vi "MegaAwesome_12_07_12a_JW.vi"() -> ()   [LabVIEW 2012]
uses:
  data/MegaAwesome_States.ctl
  <vilib>/Utility/inputDevices.llb/keyboardAcquire.vi
  <vilib>/Utility/file.llb/Read From Spreadsheet File (string).vi
  <vilib>/Utility/file.llb/Write To Spreadsheet File (string).vi
panel:
  out "Save Next?":bool
  out "Image Center X":i32
  in  "Disable Flag":bool
  out "Index":string
  in  "Slider Min":dbl=5.0
  in  "Slider Max":dbl=5.0
  out "Opj X Axis":string
  out "X Axis Display Type":string
  in  "Index-Sat":dbl=5.0
  in  "Index-Lin":dbl=5.0
  in  "IndexLog-Lin":dbl=5.0
  in  "IndexLog-Sat":dbl=5.0 caption="Num Pts"
  out "Lin Id-Log Used":dbl[](array[numeric])
  out "Lin-Vg Array-Log Used":dbl[](array[numeric])
  out "Save Array":string[][](array[string])
  out "Folder Index":i32 caption="Length"
  out "Sat Id-Used":dbl[](array[numeric])
  out "Sat Vg Array-Used":dbl[](array[numeric])
  out "Vg Array-Log-Used":dbl[](array[numeric])
  out "Sat Id-Log-Used":dbl[](array[numeric])
  out "Lin Id-Used":dbl[](array[numeric])
  out "Lin-Vg Array-Used":dbl[](array[numeric])
  out "Lin Vd":dbl
  out "Recorded Prop":T1
  out "Current State":T2
  in  "Main Tab Control":T3(tab)
  in  "Transfer File":path
  out "Transfer Folder":path
  in  "Transport\nFolder":path caption="Transport Folder"
  out "Transport\nFile":path caption="Transport File"
  in  "Image Folder":path
  out "Image File":path
  out "Fabrication Prop":T4
  out "Distances":i32[](array[numeric])
  in  "Zoom":i32(slide)=-3 scale=-5.0..5.0
  in  "Magnification":i32(ring) items=["5x", "10x", "20x", "50x", "80x"]
  in  "Undo Button":bool
  in  "Remove Button":bool
  in  "Transfer Plots":T5(tab)=enum."Saturation"
  in  "Lin-Trans Slider":dbl(slide) step=1.0 scale=-40.0..40.0 scale format="%#_1p"
  out "Sqrt-Lin":cluster{dbl[], dbl[]}[](graph)
  in  "Sat-Trans Slider":dbl(slide) step=1.0 scale=-40.0..40.0 scale format="%#_1p"
  out "Sqrt-Sat":cluster{dbl[], dbl[]}[](graph)
  out "Raw- Lin":cluster{dbl[], dbl[]}[](graph)
  out "Raw- Sat":cluster{dbl[], dbl[]}[](graph)
  in  "Log Plots":enum32{"Linear", "Saturation", "Transport"}(tab)=enum."Saturation"
  in  "Lin-Log Slider":dbl(slide) step=1.0 scale=-40.0..40.0 scale format="%#_1p"
  out "Lin-Log":cluster{dbl[], dbl[]}[](graph)
  in  "Sat-Log Slider":dbl(slide) step=1.0 scale=-40.0..40.0 scale format="%#_1p"
  out "Sat-Log":cluster{dbl[], dbl[]}[](graph)
  out "Transport":cluster{ext[], ext[]}[](graph)
  out "Transport Name:":string
  in  "Manual Controls":T6
  in  "File Controls":T7
  out "Date Recorded":string="Date Recorded" caption="Measured"
  out "Data Name:":string
  out "Image Name":string
  out "Date Created":string caption="Fabricated"
  in  "Comments:":string
  out "Rec: Length":dbl caption="Length"
  out "Rec: Width":dbl caption="Width"
  out "Rec: Dielectric (d)":dbl caption="Dielectric (d)" format="%#_3g"
  in  "New: Dielectric":dbl
  in  "New: Length":dbl
  in  "New: Width":dbl
  out "Rec: Temp":dbl caption="Sample Temp" format="%.1f"
  in  "New: Temp":dbl format="%.1f"
  out "Image Out":T8(plugin-control)
  in  "Num Pts":i32=5
  in  "Num Pts Log":i32=5 caption="Num Pts"
  out "Recorded Values Cluster":T9
  out "Calculated Values Cluster":T9 caption="Recorded Values Cluster"
  out "Re-Calculated Values Cluster":T9 caption="Recorded Values Cluster"
  in  "Independant Variable:":string(combo)="Length (um):"
  out "Image Preview":T8(plugin-control)
  out "Total Width":i32
  in  "Index Array":i32(ring) caption="Index" items=["1E", "2E", "2F", "2G", "2H", "3A", "3B", "3C", "3D", "3E", "3F", "3G", "3H", "3J", "4D", "4E", "4F", "4G", "4H", "4J", "5F", "5G", "5H", "6A", "6B", "6F", "6G", "7C", "7D", "7E", "7F", "7G", "8E", "8G", "8H", "9F", "9G", "X 1A", "X 1B", "X 1C", "X 1D", "X 1F", "X 1G", "X 2B", "X 2C", "X 2D"]
  in  "Room Temp":dbl=294.0 caption="Room Temp (K)"
  out "No Image\n File":path=path "\\\\acad1\\physics/Jurchescu-group/JW-PD/Mega Awesome/Image Not Found.png" caption="No Image File"
  out "Origin Project File":path=path "\\\\acad1\\physics/Jurchescu-group/JW-PD/Group Library/Origin Project Files/DeviceData_8_10_12a_JW.opj"
  out "No Transport\n File":path=path "\\\\acad1\\physics/Jurchescu-group/JW-PD/Mega Awesome/No Transport File.txt" caption="No Transport File"
  in  "Transport Style Controls":T10={"Transport Line Size"=1, "Transport Line Color"=16772608} {"Transport Line Size" items=["Extra Small", "Small", "Medium", "Large", "Extra Large"]}
  out "Application Directory":path
  out "Progress":i32(slide) max=46 step=1 scale=0.0..100.0
  # "1)  Select the Transfer File that you would like to analyze:"
  # "Transfer Location"
  # "2) What else would you like to view during your analysis?"
  # "Transport Location"
  # "Image Location"
  # "Recorded"
  # "Calculated"
  # "Re-Calculated"
  # "Manual"
  # "um"
  # "V"
  # "V"
  # "V"
  # "Default File Choices"
  # "Default Analysis Values"
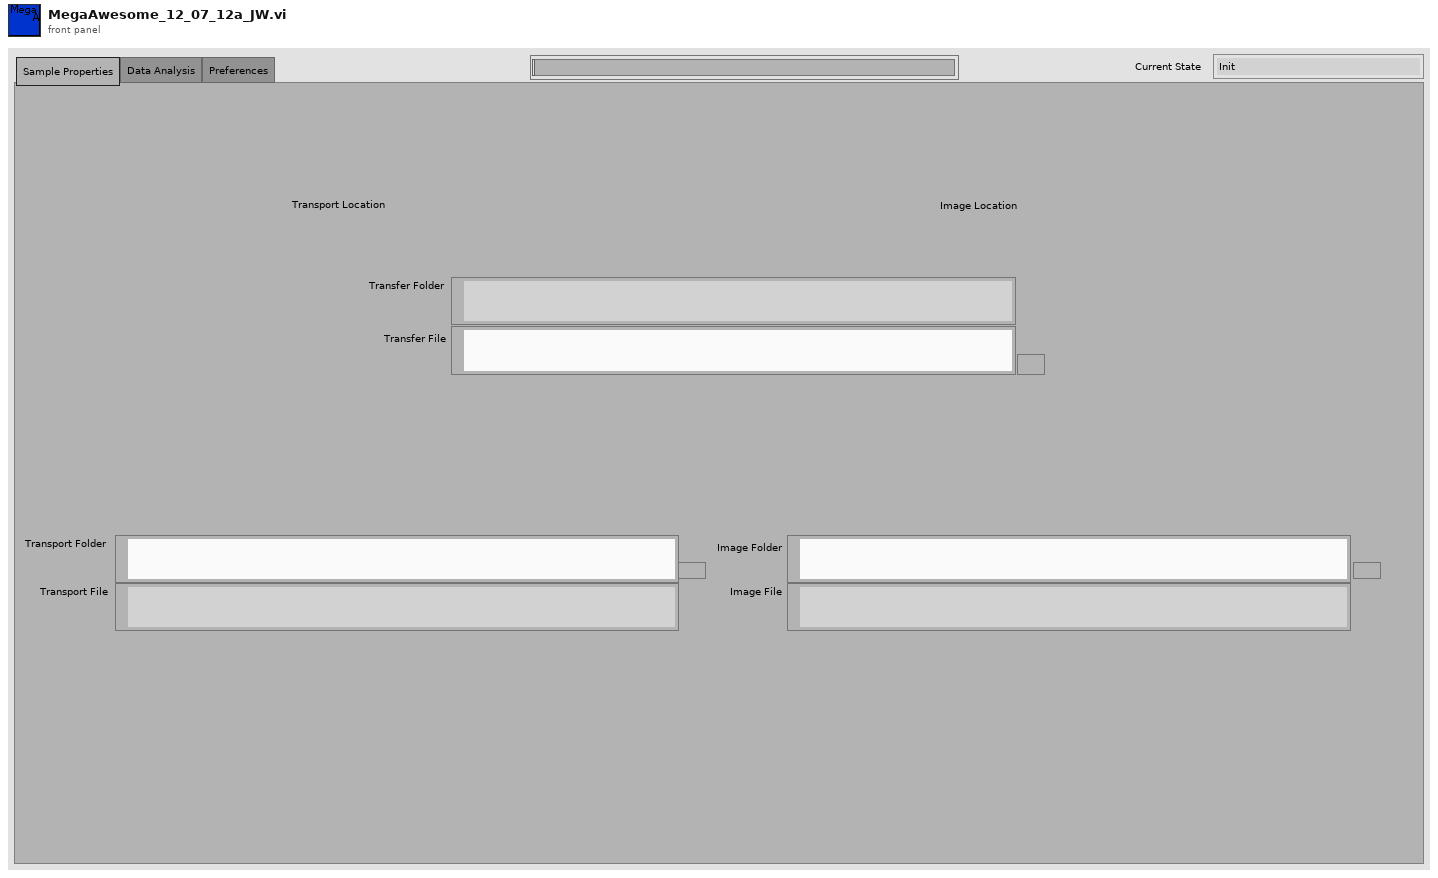
[diagram p1: front panel]
types:
  T1 = cluster{"Date Recorded":string, "Index":string, "Length":dbl, "Width":dbl, "Sample Temp":dbl}
  T2 = typedef "MegaAwesome_States.ctl" = enum16{"Init", "File Missing", "No Event", "Read Data", "Calculated Values", "Re-Calculated Values", "Next File", "Previous File", "Discard File", "Save", "Save Lines", "Export", "Exit"}
  T3 = enum32{"Sample Properties", "Data Analysis", "Preferences"}
  T4 = cluster{"Date Created":string, "Material":string, "Solvent":string, "Concentration":dbl, "Method":string, "Dielectric (nm)":dbl, "Treatment":string, "Comments":string}
  T5 = enum32{"Linear", "Saturation", "Raw-Linear", "Raw-Saturation"}
  T6 = cluster{"Manual-Temp":bool, "Manual-Width":bool, "Manuel-Length":bool, "Manuel-Dielectric":bool, "Manual Comments":bool}
  T7 = cluster{"Previous File":bool, "Discard ":bool, "Save Lines":bool, "Close":bool, "Next File ":bool, "Save":bool, "Save Next":bool, "Export":bool}
  T8 = typedef "IMAQ Image.ctl" = refnum<image>
  T9 = cluster{"Mobility-Sat":dbl, "Moblitity-Lin":dbl, "On/Off":dbl, "Off Current":dbl, "Vt-Sat":dbl, "STS":dbl, "Trap Density-VT":dbl, "Trap Density-STS":dbl}
  T10 = cluster{"Transport Line Size":u16, "Transport Line Color":u32}
  T11 = enum8{"Enabled", "Disabled", "Disabled and Grayed Out"}
  T12 = typedef "LVBoundsTypeDef.ctl" = cluster{"Width":u32, "Height":u32}
  T13 = enum16{"0", "1", "2", "3", "4", "5", "6", "7", "8", "9", "A", "B", "C", "D", "E", "F", "G", "H", "I", "J", "K", "L", "M", "N", "O", "P", "Q", "R", "S", "T", "U", "V", "W", "X", "Y", "Z", "F1", "F2", "F3", "F4", "F5", "F6", "F7", "F8", "F9", "F10", "F11", "F12", "F13", "F14", "F15", "ADD", "BACK", "BACKSLASH", "CAPITAL", "COMMA", "DECIMAL", "DELETE", "DIVIDE", "DOWN", "END", "EQUALS", "ESCAPE", "GRAVE (`)", "HOME", "INSERT", "LBRACKET", "LCONTROL", "LEFT", "L ALT", "LSHIFT", "LWIN", "MINUS", "MULTIPLY", "NEXT", "NUMLOCK", "NUMPAD_0", "NUMPAD_1", "NUMPAD_2", "NUMPAD_3", "NUMPAD_4", "NUMPAD_5", "NUMPAD_6", "NUMPAD_7", "NUMPAD_8", "NUMPAD_9", "PAUSE", "PERIOD", "PRIOR (PG UP)", "RBRACKET", "RCONTROL", "RETURN", "RIGHT", "R ALT", "RSHIFT", "RWIN", "SCROLL", "SEMICOLON", "SLASH", "SPACE", "SUBTRACT", "TAB", "UP", "ENTER (num pad)", "' (quote)"}[]
  T14 = enum16{"0", "1", "2", "3", "4", "5", "6", "7", "8", "9", "A", "B", "C", "D", "E", "F", "G", "H", "I", "J", "K", "L", "M", "N", "O", "P", "Q", "R", "S", "T", "U", "V", "W", "X", "Y", "Z", "F1", "F2", "F3", "F4", "F5", "F6", "F7", "F8", "F9", "F10", "F11", "F12", "F13", "F14", "F15", "ADD", "BACK", "BACKSLASH", "CAPITAL", "COMMA", "DECIMAL", "DELETE", "DIVIDE", "DOWN", "END", "EQUALS", "ESCAPE", "GRAVE (`)", "HOME", "INSERT", "LBRACKET", "LCONTROL", "LEFT", "L ALT", "LSHIFT", "LWIN", "MINUS", "MULTIPLY", "NEXT", "NUMLOCK", "NUMPAD_0", "NUMPAD_1", "NUMPAD_2", "NUMPAD_3", "NUMPAD_4", "NUMPAD_5", "NUMPAD_6", "NUMPAD_7", "NUMPAD_8", "NUMPAD_9", "PAUSE", "PERIOD", "PRIOR (PG UP)", "RBRACKET", "RCONTROL", "RETURN", "RIGHT", "R ALT", "RSHIFT", "RWIN", "SCROLL", "SEMICOLON", "SLASH", "SPACE", "SUBTRACT", "TAB", "UP", "ENTER (num pad)", "' (quote)"}
  T15 = typedef "ROI Descriptor" = cluster{"Global Rectangle":i32[], "Contours":cluster{"ID":enum32{"External", "Internal"}, "Type":u32, "Coordinates":i32[]}[]}
  T16 = cluster{string, sgl, bool, bool, bool, bool, bool, bool, i32}
  T17 = cluster{i32, cluster{string, sgl, bool, bool, bool, bool, bool, bool, i32}, i32, i32}
  T18 = cluster{"Global Rectangle":i32[], "Contours":cluster{"Contour Type":u32, "ROI Type":u32, "Points":i32[]}[]}
  T19 = cluster{"Contour Type":u32, "ROI Type":u32, "Points":i32[]}[]
  T20 = cluster{"[0]":cluster{dbl[], dbl[]}, "[1]":cluster{dbl[], dbl[]}, "[2]":cluster{dbl[], dbl[]}, "[3]":cluster{dbl[], dbl[]}, "[4]":cluster{dbl[], dbl[]}, "[5]":cluster{dbl[], dbl[]}, "[6]":cluster{dbl[], dbl[]}, "[7]":cluster{dbl[], dbl[]}, "[8]":cluster{dbl[], dbl[]}}
  T21 = cluster{i32[], cluster{"Contour Type":u32, "ROI Type":u32, "Points":i32[]}[]}
  T22 = cluster{"Contour Type":u32, "ROI Type":u32, "Points":i32[]}
  T23 = cluster{"Points[0]":i32, "Points[1]":i32, "Points[2]":i32, "Points[3]":i32, "Points[4]":i32, "Points[5]":i32, "Points[6]":i32, "Points[7]":i32, "Points[8]":i32}
  T24 = cluster{"Sat Vg Used":dbl[], "Sat Sqrt(Id) Used ":dbl[], "Lin Vg Used":dbl[], "Lin Sqrt(Id) Used":dbl[], "Index-Lin":dbl, "Index-Sat":dbl}
  T25 = cluster{"Raw Sat":cluster{dbl[], dbl[]}[], "Sqrt Sat":cluster{dbl[], dbl[]}[], "Log Sat":cluster{dbl[], dbl[]}[], "Raw Lin":cluster{dbl[], dbl[]}[], "Sqrt Lin":cluster{dbl[], dbl[]}[], "Log Lin":cluster{dbl[], dbl[]}[]}
  T26 = cluster{"Mobility-Sat":dbl, "Vt-Sat":dbl, "Mobility-Lin":dbl, "Vt-Lin":dbl, "Off I-Sat":dbl, "On/Off I-Sat":dbl}
  T27 = cluster{"Sat Vg Used":dbl[], "Sat Log(Id) Used":dbl[], "Lin Vg Used":dbl[], "Lin Log(Id) Used":dbl[], "STS Index-Sat":dbl, "STS Index-Lin":dbl}
  T28 = cluster{"Independant  Variable Indicator":string, "Parameter String Indicator":string}
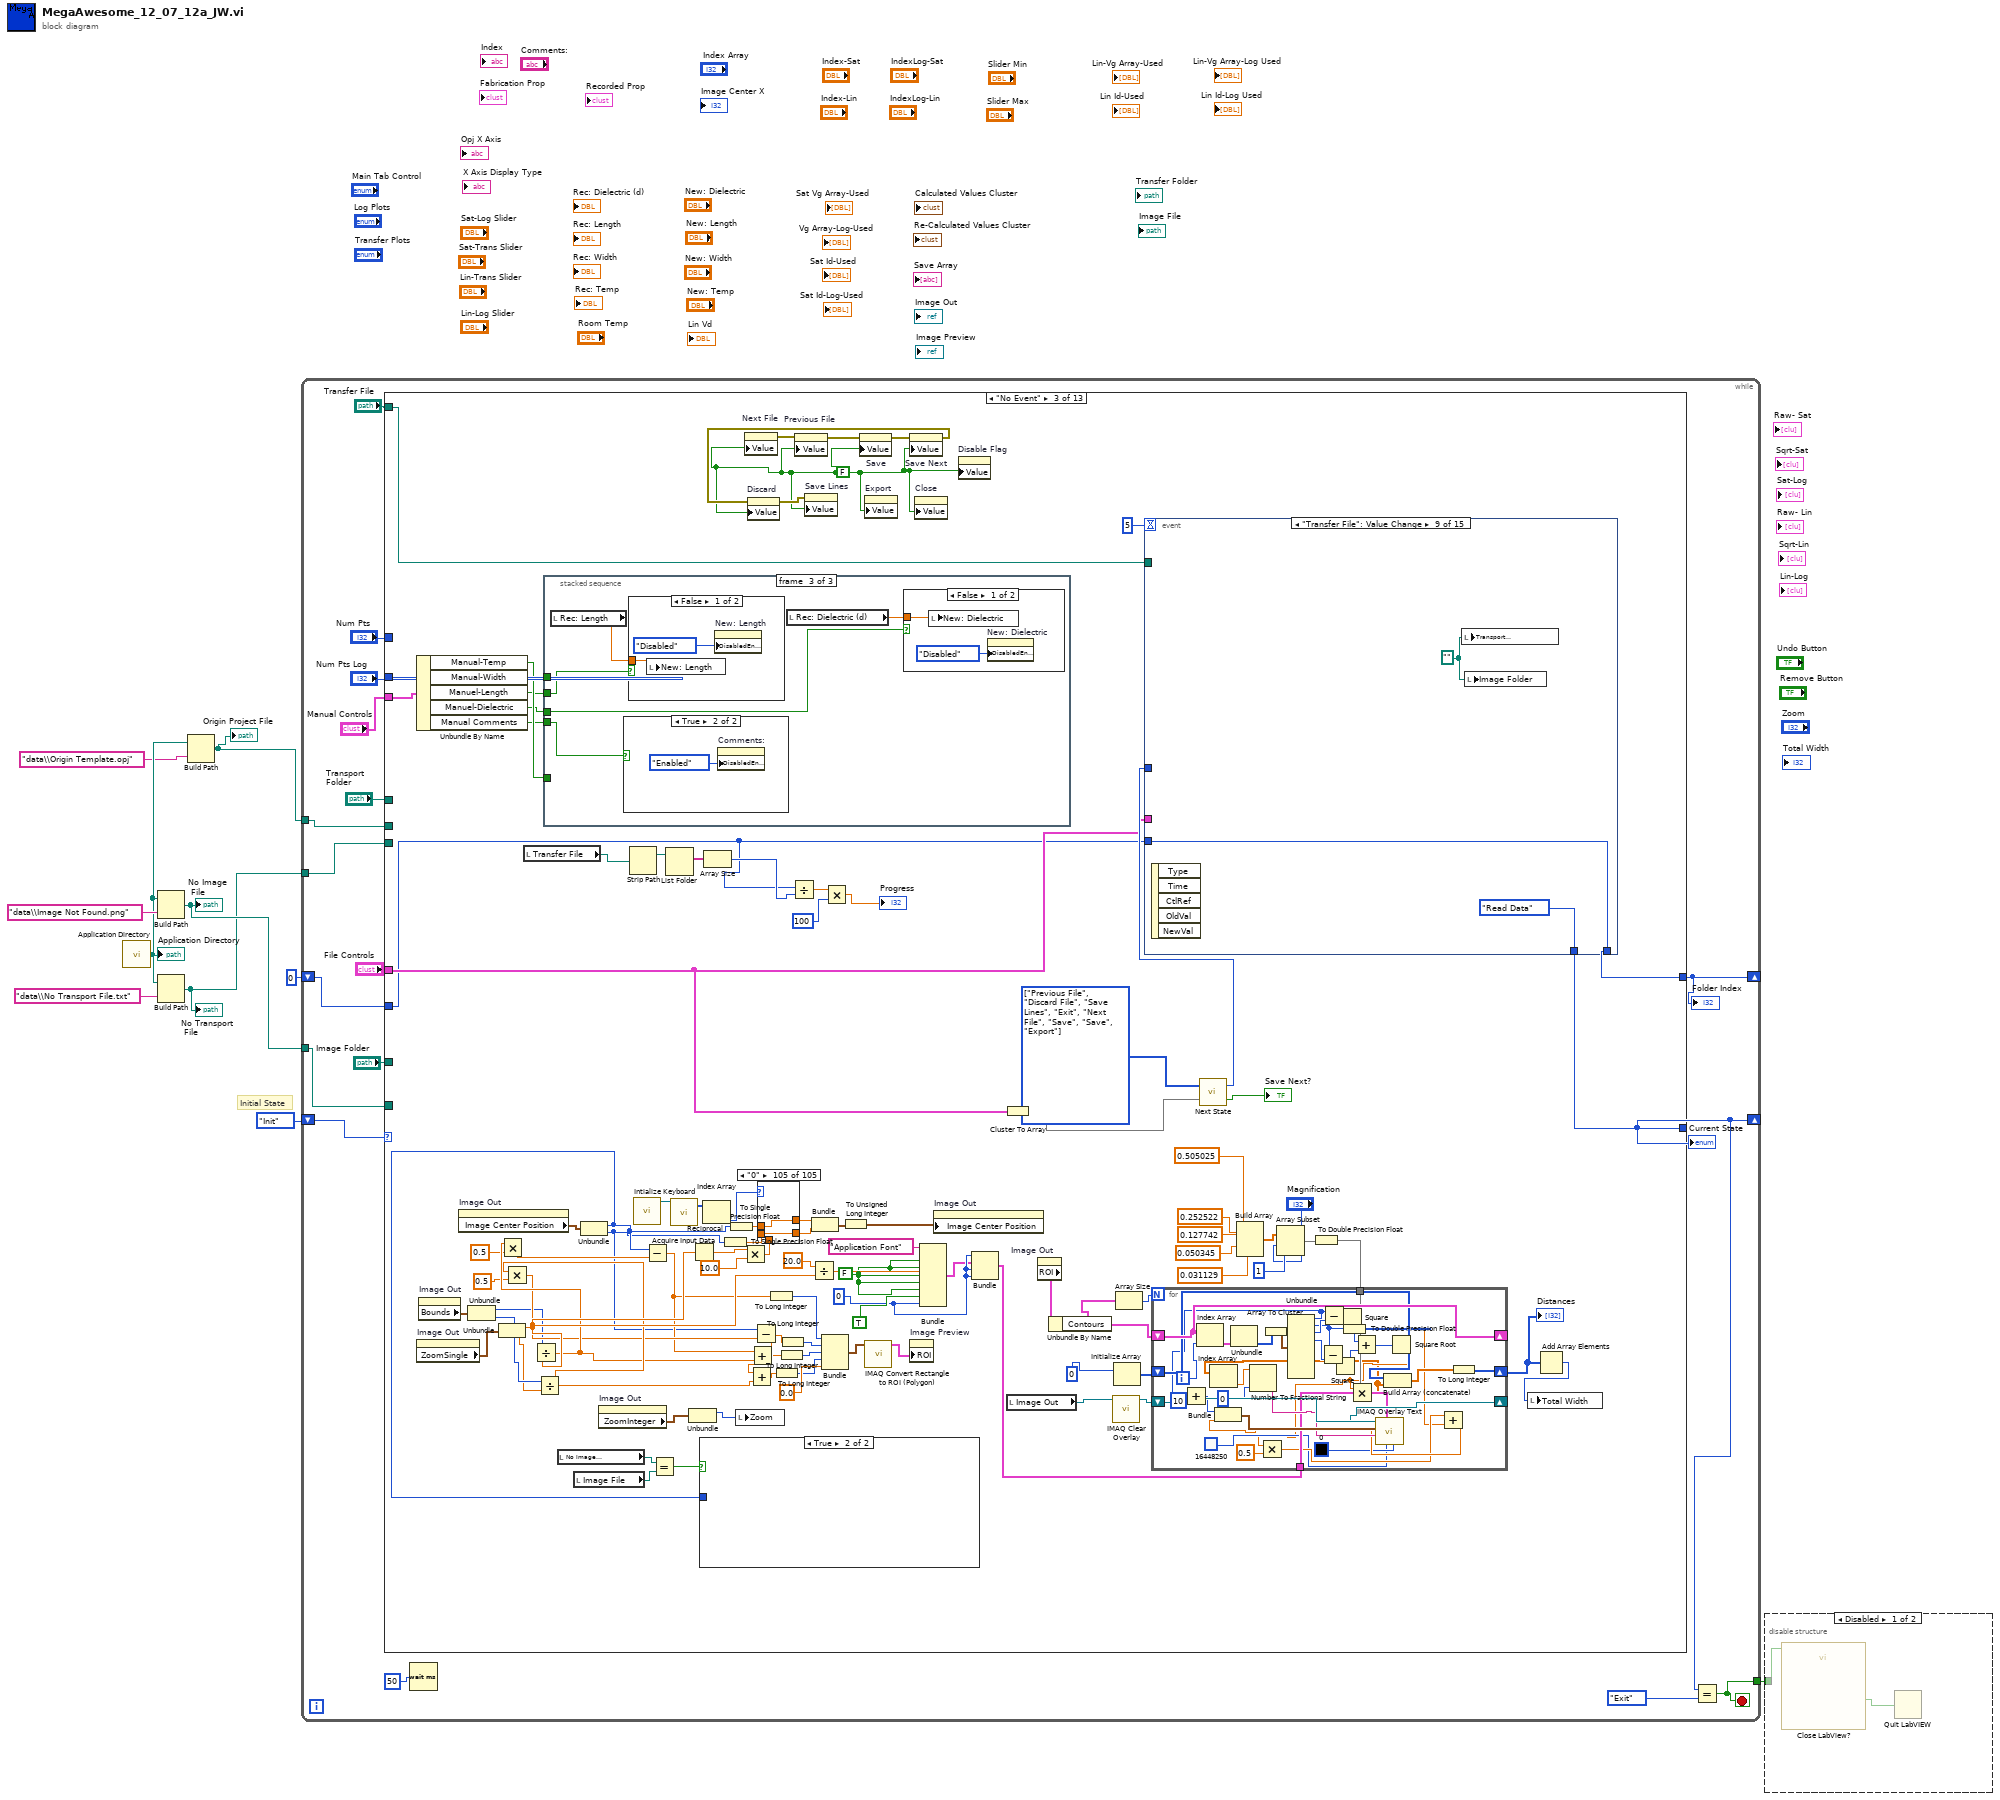
[diagram p0: block diagram]
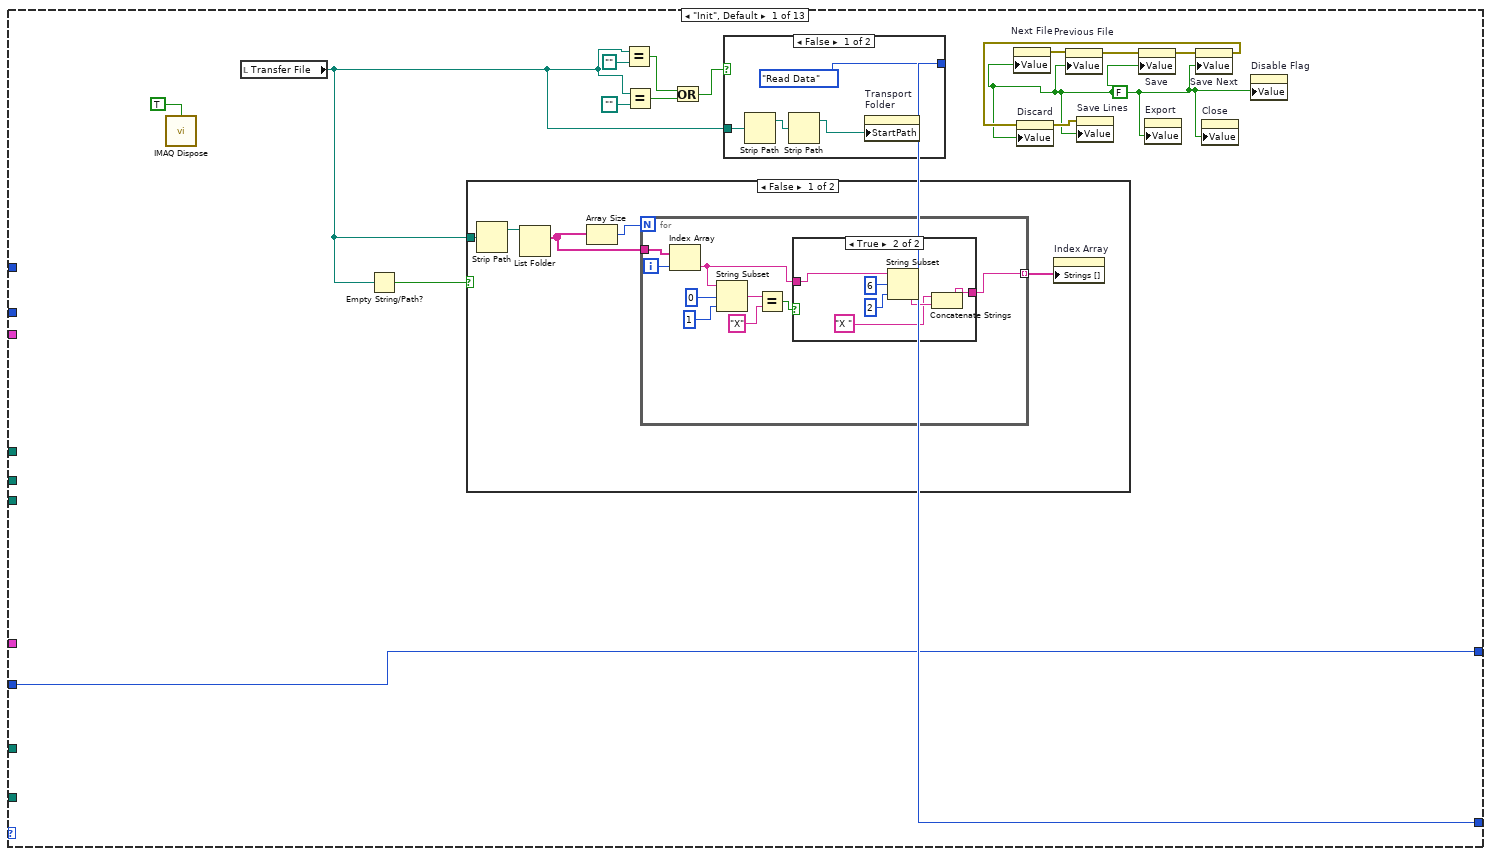
[diagram p3: hidden frame]
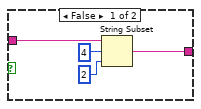
[diagram p4: hidden frame]
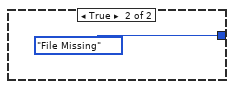
[diagram p6: hidden frame]
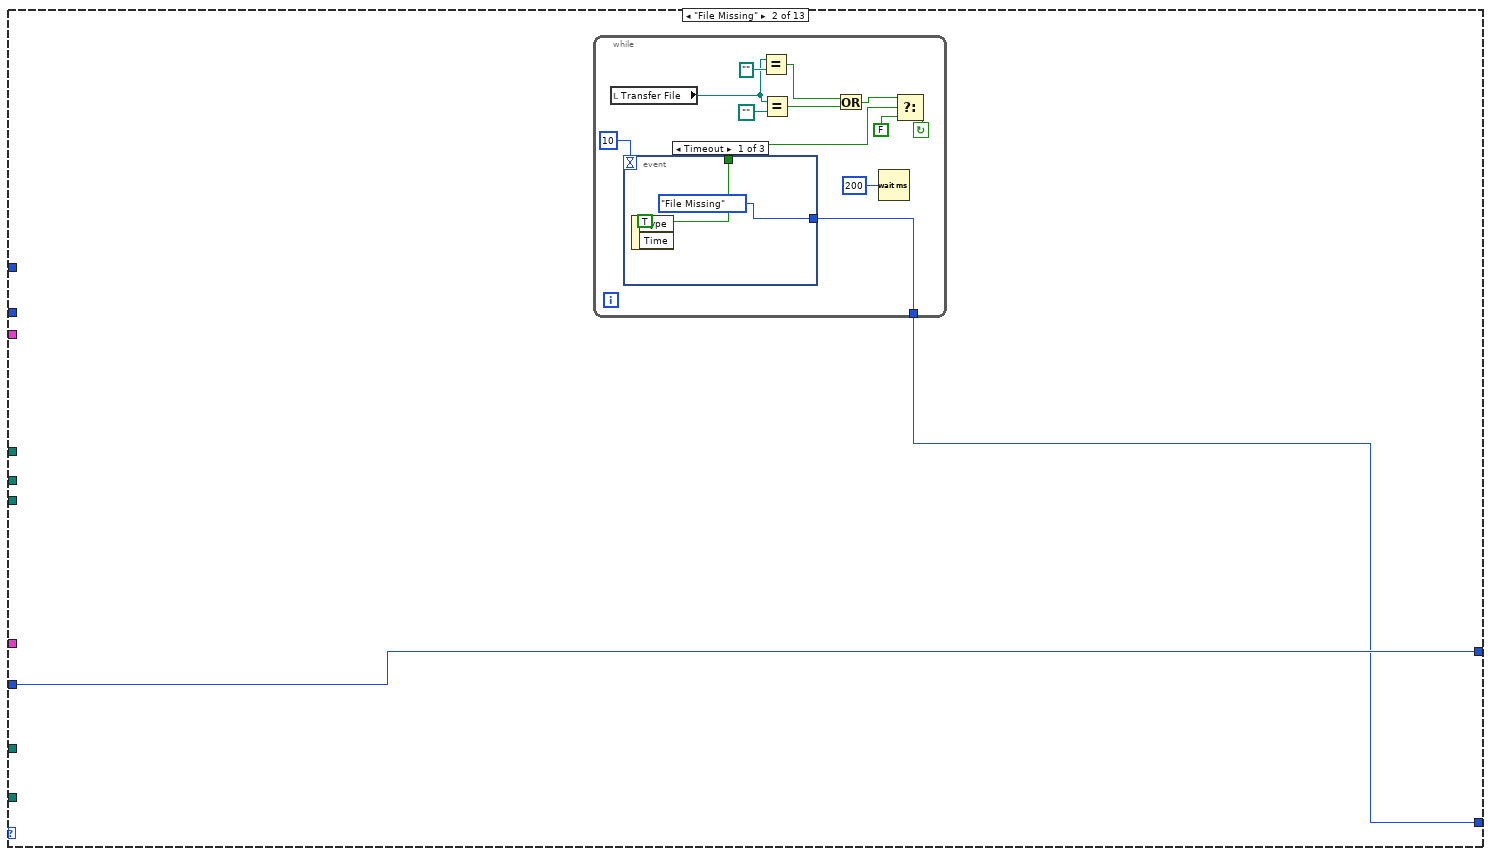
[diagram p7: hidden frame]
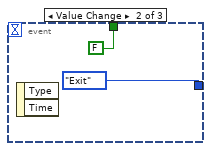
[diagram p8: hidden frame]
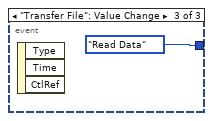
[diagram p9: hidden frame]
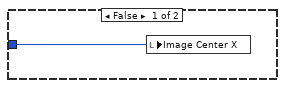
[diagram p10: hidden frame]
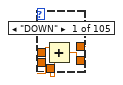
[diagram p11: hidden frame]
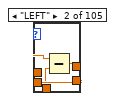
[diagram p12: hidden frame]
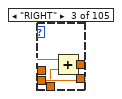
[diagram p13: hidden frame]
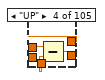
[diagram p14: hidden frame]
diagram:
  # "Initial State"
  n1 = call <vilib>:"Application Directory.vi"() -> ("Application Directory"=w3:path)
  "Application Directory" <- w3
  n2 = Build Path(base path=w3, name or relative path="data\\Image Not Found.png") -> (appended path=w6:path)
  "No Image\n File" <- w6
  n3 = Build Path(base path=w3, name or relative path="data\\No Transport File.txt") -> (appended path=w5:path)
  "No Transport\n File" <- w5
  n4 = Build Path(base path=w3, name or relative path="data\\Origin Template.opj") -> (appended path=w4:path)
  "Origin Project File" <- w4
  n5 = while {
    shift-right: [w12] -> _
    shift-left: MegaAwesome_States."Init" -> [w14]
    shift-right: [w11] -> _
    shift-left: 0 -> [w22]
    tunnel: w6 -> [w19]
    tunnel: w5 -> [w17]
    tunnel: w4 -> [w16]
    tunnel: [w15] -> w1
    stop <- w15 stop-if-true
    n6 = case shown="\"No Event\"" w14 {
      tunnel: [w30 w73 w181 MegaAwesome_States."Calculated Values" MegaAwesome_States."Re-Calculated Values" MegaAwesome_States."No Event" MegaAwesome_States."Read Data" MegaAwesome_States."Read Data" MegaAwesome_States."Init" w836 MegaAwesome_States."Exit" MegaAwesome_States."No Event" MegaAwesome_States."No Event"] -> w12
      tunnel: "Transfer File" -> [_ _ w173 w634 w682 _ w783 w794 w821 w841 _ _ _]
      tunnel: "Num Pts" -> [_ _ _ _ w717 _ _ _ _ _ _ _ _]
      tunnel: "Num Pts Log" -> [_ _ _ _ w716 _ _ _ _ _ _ _ _]
      tunnel: "Image Folder" -> [_ _ _ _ w713 _ _ _ _ _ _ w1356 _]
      tunnel: w19 -> [_ _ _ _ w712 _ _ _ _ _ _ _ _]
      tunnel: [w28 w74 w174 w639 w711 w743 w769 w792 w810 w842 w1342 w1366 w1372] -> w11
      tunnel: w22 -> [w28 w74 w92 w637 w711 w743 w770 w793 _ w842 w1342 w1366 w1372]
      tunnel: "Manual Controls" -> [_ _ w183 _ _ _ _ _ _ w840 _ _ _]
      tunnel: "File Controls" -> [_ _ w171 _ _ _ _ _ _ _ _ _ _]
      tunnel: "Transport\nFolder" -> [_ _ _ _ w678 _ _ _ _ _ _ _ _]
      tunnel: w17 -> [_ _ _ _ w677 _ _ _ _ _ _ _ _]
      tunnel: w16 -> [_ _ _ _ _ _ _ _ _ _ _ _ w1371]
      frame "Init", Default {
        w31 = FALSE
        n7 = call "IMAQ Dispose"("All Images? (No)"=TRUE) -> ()  [unwired: 5 in, 1 out]
        n8 = local read "Transfer File"() -> (w29:path)
        n9 = Empty String/Path?(string/path=w29) -> (empty?=w38:bool)
        n10 = case shown="False" w38 {
          tunnel: w29 -> [w45 _]
          frame False {
            n11 = Strip Path(path=w45) -> (stripped path=w47:path)  [unwired: 1 out]
            n12 = List Folder(path=w47) -> (filenames=w46:string[])  [unwired: 3 in, 3 out]
            n13 = Array Size(array=w46) -> (size(s)=w48:i32)
            n14 = for {
              N: w48 -> [_]
              tunnel: w46 -> [w57]
              tunnel: [w55] -> w44 mode=indexing
              i -> [w56]
              n15 = Index Array(array=w57, index=w56) -> (element=w54:string)
              n16 = String Subset(string=w54, offset (0)=0, length (rest)=1) -> (substring=w51:string)
              n17 = Equal?(x=w51, y="X") -> (x = y?=w50:bool)
              n18 = case shown="True" w50 {
                tunnel: w54 -> [w61 w65]
                tunnel: [w58 w64] -> w55
                frame False {
                  n19 = String Subset(string=w61, offset (0)=4, length (rest)=2) -> (substring=w58:string)
                }
                frame True {
                  n20 = String Subset(string=w65, offset (0)=6, length (rest)=2) -> (substring=w63:string)
                  n21 = Concatenate Strings("X ", w63) -> (w64:string)
                }
              }
            }
            n22 = property on="Index Array" class="Ring (strict)"("Strings []"=w44) -> ()  [unwired: 2 in, 2 out]
          }
          frame True {
          }
        }
        n23 = Equal?(x=w29, y=path "") -> (x = y?=w41:bool)
        n24 = Equal?(x=w29, y=path "") -> (x = y?=w40:bool)
        n25 = Or(x=w41, y=w40) -> (x .or. y?=w43:bool)
        n26 = case shown="False" w43 {
          tunnel: [MegaAwesome_States."Read Data" MegaAwesome_States."File Missing"] -> w30
          tunnel: w29 -> [w70 _]
          frame False {
            n27 = Strip Path(path=w70) -> (stripped path=w69:path)  [unwired: 1 out]
            n28 = Strip Path(path=w69) -> (stripped path=w68:path)  [unwired: 1 out]
            n29 = property on="Transport\nFolder" class="Path"("StartPath"=w68) -> ()  [unwired: 2 in, 2 out]
          }
          frame True {
          }
        }
        n30 = property on="Next File" class="Bool (strict)"("Value"=w31) -> (error out=w36:errorcluster)  [unwired: 2 in, 1 out]
        n31 = property on="Previous File" class="Bool (strict)"(error in=w36, "Value"=w31) -> (error out=w35:errorcluster)  [unwired: 1 in, 1 out]
        n32 = property on="Save" class="Bool (strict)"(error in=w35, "Value"=w31) -> (error out=w34:errorcluster)  [unwired: 1 in, 1 out]
        n33 = property on="Export" class="Bool (strict)"("Value"=w31) -> ()  [unwired: 2 in, 2 out]
        n34 = property on="Save Next" class="Bool (strict)"(error in=w34, "Value"=w31) -> (error out=w33:errorcluster)  [unwired: 1 in, 1 out]
        n35 = property on="Discard" class="Bool (strict)"(error in=w33, "Value"=w31) -> (error out=w32:errorcluster)  [unwired: 1 in, 1 out]
        n36 = property on="Save Lines" class="Bool (strict)"(error in=w32, "Value"=w31) -> ()  [unwired: 1 in, 2 out]
        n37 = property on="Close" class="Bool (strict)"("Value"=w31) -> ()  [unwired: 2 in, 2 out]
        n38 = property on="Disable Flag" class="Bool (strict)"("Value"=w31) -> ()  [unwired: 2 in, 2 out]
      }
      frame "File Missing" {
        n39 = while {
          tunnel: [w81] -> w73
          stop <- w77 continue-if-true
          n40 = local read "Transfer File"() -> (w82:path)
          n41 = event shown="[0] Timeout" {
            selector: _ -> [_ _ _]
            dyn-events: _ -> [_ _ _]
            timeout: 10 -> [_ _ _]
            tunnel: [MegaAwesome_States."File Missing" MegaAwesome_States."Exit" MegaAwesome_States."Read Data"] -> w81
            tunnel: [TRUE FALSE _] -> w80
            event Timeout {
              n42 = event-data() -> ()  [unwired: 1 in, 2 out]
            }
            event "File Controls.Close": Value Change {
              n43 = event-data() -> ()  [unwired: 1 in, 2 out]
            }
            event "Transfer File": Value Change {
              n44 = event-data() -> ()  [unwired: 1 in, 3 out]
            }
          }
          n45 = Equal?(x=w82, y=path "") -> (x = y?=w84:bool)
          n46 = Equal?(x=w82, y=path "") -> (x = y?=w85:bool)
          n47 = Or(x=w84, y=w85) -> (x .or. y?=w79:bool)
          n48 = Wait (ms)(milliseconds to wait=u32 200) -> ()  [unwired: 1 out]
          n49 = Select(t=w79, s=w80, f=FALSE) -> (s? t:f=w77:bool)
        }
      }
      frame "No Event" {
        w162 = FALSE
        w164 = 0
        w172 = FALSE
        w190 = T2[] [enum."Previous File", enum."Discard File", enum."Save Lines", enum."Exit", enum."Next File", enum."Save", enum."Save", enum."Export"] items=["Init", "File Missing", "No Event", "Read Data", "Calculated Values", "Re-Calculated Values", "Next File", "Previous File", "Discard File", "Save", "Save Lines", "Export", "Exit"]
        n50 = Unbundle By Name(w183) -> ("Manual-Temp"=w188:bool, "Manual-Width"=w187:bool, "Manuel-Length"=w186:bool, "Manuel-Dielectric"=w185:bool, "Manual Comments"=w184:bool)
        n51 = property on="Image Out" class="ImageControl"() -> ("ZoomSingle"=w151:cluster{"X":sgl, "Y":sgl})  [unwired: 2 in, 2 out]
        n52 = property on="Image Out" class="ImageControl"() -> ("Bounds"=w150:T12)  [unwired: 2 in, 2 out]
        n53 = property on="Image Out" class="ImageControl"() -> ("Image Center Position"=w147:cluster{"X":u32, "Y":u32})  [unwired: 2 in, 2 out]
        n54 = Unbundle(w150) -> ("Width"=w153:u32, "Height"=w154:u32)
        n55 = Unbundle(w151) -> ("X"=w168:sgl, "Y"=w152:sgl)
        n56 = local read "Transfer File"() -> (w95:path)
        n57 = Divide(x=w153, y=w168) -> (x/y=w159:sgl)
        n58 = Multiply(x=w159, y=sgl 0.5) -> (x*y=w157:sgl)
        n59 = Divide(x=w154, y=w152) -> (x/y=w160:sgl)
        n60 = Multiply(x=w160, y=sgl 0.5) -> (x*y=w158:sgl)
        n61 = stacked-sequence {
          tunnel: w188 -> [w592 _ _]
          tunnel: w187 -> [_ w606 _]
          tunnel: w186 -> [_ _ w619]
          tunnel: w185 -> [_ _ w617]
          tunnel: w184 -> [_ _ w616]
          frame #0 {
            n62 = local read "Rec: Temp"() -> (w591:dbl)
            n63 = case shown="True" w592 {
              tunnel: w591 -> [w597 _]
              frame False {
                n64 = local read "Rec: Temp"() -> (w595:dbl)
                n65 = property on="New: Temp" class="DigNum (strict)"("DisabledEnum"=T11."Disabled" ("Disabled")) -> ()  [unwired: 2 in, 2 out]
                n66 = Equal To 0?(x=w595) -> (x = 0?=w596:bool)
                n67 = local write "New: Temp"(w597) -> ()
                n68 = case shown="True" w596 {
                  tunnel: [w598 w599] -> w593
                  tunnel: w595 -> [w598 _]
                  frame False {
                  }
                  frame True {
                    n69 = local read "Room Temp"() -> (w599:dbl)
                  }
                }
                n70 = local write "Rec: Temp"(w593) -> ()
                n71 = local write "New: Temp"(w593) -> ()
              }
              frame True {
                n72 = property on="New: Temp" class="DigNum (strict)"("DisabledEnum"=T11."Enabled" ("Disabled")) -> ()  [unwired: 2 in, 2 out]
              }
            }
          }
          frame #1 {
            n73 = local read "New: Width"() -> (w607:dbl)
            n74 = local read "Total Width"() -> (w603:i32)
            n75 = case shown="False" w606 {
              frame False {
                n76 = property on="New: Width" class="DigNum (strict)"("DisabledEnum"=T11."Disabled" ("Disabled")) -> ()  [unwired: 2 in, 2 out]
              }
              frame True {
                n77 = property on="New: Width" class="DigNum (strict)"("DisabledEnum"=T11."Enabled" ("Disabled")) -> ()  [unwired: 2 in, 2 out]
              }
            }
            n78 = Not(x=w606) -> (.not. x?=w601:bool)
            n79 = Not Equal?(x=w603, y=w607) -> (x != y?=w602:bool)
            n80 = Equal To 0?(x=w603) -> (x = 0?=w605:bool)
            n81 = And(x=w601, y=w605) -> (x .and. y?=w604:bool)
            n82 = case shown="False" w604 {
              tunnel: w603 -> [w611 _]
              tunnel: w602 -> [w610 _]
              tunnel: w601 -> [w609 _]
              frame False {
                n83 = And(x=w609, y=w610) -> (x .and. y?=w608:bool)
                n84 = case shown="True" w608 {
                  tunnel: w611 -> [_ w612]
                  frame False {
                  }
                  frame True {
                    n85 = property on="New: Width" class="DigNum (strict)"("Val(Sgnl)"=w612) -> ()  [unwired: 2 in, 2 out]
                  }
                }
              }
              frame True {
                n86 = local read "Rec: Width"() -> (w613:dbl)
                n87 = local write "New: Width"(w613) -> ()
              }
            }
          }
          frame #2 {
            n88 = local read "Rec: Length"() -> (w620:dbl)
            n89 = case shown="True" w616 {
              frame False {
                n90 = property on="Comments:" class="Str"("DisabledEnum"=T11."Disabled" ("Disabled")) -> ()  [unwired: 2 in, 2 out]
              }
              frame True {
                n91 = property on="Comments:" class="Str"("DisabledEnum"=T11."Enabled" ("Disabled")) -> ()  [unwired: 2 in, 2 out]
              }
            }
            n92 = case shown="False" w619 {
              tunnel: w620 -> [w627 _]
              frame False {
                n93 = local write "New: Length"(w627) -> ()
                n94 = property on="New: Length" class="DigNum (strict)"("DisabledEnum"=T11."Disabled" ("Disabled")) -> ()  [unwired: 2 in, 2 out]
              }
              frame True {
                n95 = property on="New: Length" class="DigNum (strict)"("DisabledEnum"=T11."Enabled" ("Disabled")) -> ()  [unwired: 2 in, 2 out]
              }
            }
            n96 = local read "Rec: Dielectric (d)"() -> (w618:dbl)
            n97 = case shown="False" w617 {
              tunnel: w618 -> [w624 _]
              frame False {
                n98 = local write "New: Dielectric"(w624) -> ()
                n99 = property on="New: Dielectric" class="DigNum (strict)"("DisabledEnum"=T11."Disabled" ("Disabled")) -> ()  [unwired: 2 in, 2 out]
              }
              frame True {
                n100 = property on="New: Dielectric" class="DigNum (strict)"("DisabledEnum"=T11."Enabled" ("Disabled")) -> ()  [unwired: 2 in, 2 out]
              }
            }
          }
        }
        n101 = local read "No Image\n File"() -> (w121:path)
        n102 = local read "Image File"() -> (w120:path)
        n103 = Unbundle(w147) -> ("X"=w102:u32, "Y"=w100:u32)
        n104 = property on="Image Out" class="ImageControl"() -> ("ZoomInteger"=w124:cluster{"X":i32, "Y":i32})  [unwired: 2 in, 2 out]
        n105 = Strip Path(path=w95) -> (stripped path=w99:path)  [unwired: 1 out]
        n106 = call <vilib>:"Intialize Keyboard.vi"() -> ("device ID"=w145:refnum<k1>)  [unwired: 10 in, 1 out]
        n107 = Subtract(x=w102, y=w157) -> (x-y=w110:sgl)
        n108 = Equal?(x=w121, y=w120) -> (x = y?=w119:bool)
        n109 = List Folder(path=w99) -> (filenames=w98:string[])  [unwired: 3 in, 3 out]
        n110 = call-poly <vilib>:"Acquire Input Data.vi"("device ID"=w145) -> ("keys pressed"=w146:T13)  [unwired: 16 in, 2 out]
        n111 = Unbundle(w124) -> ("X"=w123:i32)  [unwired: 1 out]
        n112 = Reciprocal(x=w168) -> (1/x=w169:sgl)
        n113 = case shown="True" w119 {
          tunnel: w102 -> [w191 _]
          frame False {
            n114 = local write "Image Center X"(w191) -> ()
          }
          frame True {
          }
        }
        n115 = Index Array(array=w146) -> (element=w104:T14)  [unwired: 1 in]
        n116 = Array Size(array=w98) -> (size(s)=w94:i32)
        n117 = To Single Precision Float(number=w100) -> (single precision float=w101:sgl)
        n118 = To Single Precision Float(number=w102) -> (single precision float=w103:sgl)
        n119 = local write "Zoom"(w123) -> ()
        n120 = Multiply(x=w169, y=sgl 10.0) -> (x*y=w167:sgl)
        n121 = property on="Next File" class="Bool (strict)"("Value"=w172) -> (error out=w179:errorcluster)  [unwired: 2 in, 1 out]
        n122 = Add(x=w110, y=w159) -> (x+y=w108:sgl)
        n123 = Subtract(x=w100, y=w158) -> (x-y=w112:sgl)
        n124 = Add(x=w112, y=w160) -> (x+y=w106:sgl)
        n125 = case shown="\"0\"" w104 {
          tunnel: w103 -> [w228 w234 w238 w240 w244 w246 w248 w250 w252 w254 w256 w258 w260 w262 w264 w266 w268 w270 w272 w274 w276 w278 w280 w282 w284 w286 w288 w290 w292 w294 w296 w298 w300 w302 w304 w306 w308 w310 w312 w314 w316 w318 w320 w322 w324 w326 w328 w330 w332 w334 w336 w338 w340 w342 w344 w346 w348 w350 w352 w354 w356 w358 w360 w362 w364 w366 w368 w370 w372 w374 w376 w378 w380 w382 w384 w386 w388 w390 w392 w394 w396 w398 w400 w402 w404 w406 w408 w410 w412 w414 w416 w418 w420 w422 w424 w426 w428 w430 w432 w434 w436 w438 w440 w442 w444]
          tunnel: [w228 w233 w237 w240 w244 w246 w248 w250 w252 w254 w256 w258 w260 w262 w264 w266 w268 w270 w272 w274 w276 w278 w280 w282 w284 w286 w288 w290 w292 w294 w296 w298 w300 w302 w304 w306 w308 w310 w312 w314 w316 w318 w320 w322 w324 w326 w328 w330 w332 w334 w336 w338 w340 w342 w344 w346 w348 w350 w352 w354 w356 w358 w360 w362 w364 w366 w368 w370 w372 w374 w376 w378 w380 w382 w384 w386 w388 w390 w392 w394 w396 w398 w400 w402 w404 w406 w408 w410 w412 w414 w416 w418 w420 w422 w424 w426 w428 w430 w432 w434 w436 w438 w440 w442 w444] -> w143
          tunnel: w101 -> [w230 w232 w236 w242 w243 w245 w247 w249 w251 w253 w255 w257 w259 w261 w263 w265 w267 w269 w271 w273 w275 w277 w279 w281 w283 w285 w287 w289 w291 w293 w295 w297 w299 w301 w303 w305 w307 w309 w311 w313 w315 w317 w319 w321 w323 w325 w327 w329 w331 w333 w335 w337 w339 w341 w343 w345 w347 w349 w351 w353 w355 w357 w359 w361 w363 w365 w367 w369 w371 w373 w375 w377 w379 w381 w383 w385 w387 w389 w391 w393 w395 w397 w399 w401 w403 w405 w407 w409 w411 w413 w415 w417 w419 w421 w423 w425 w427 w429 w431 w433 w435 w437 w439 w441 w443]
          tunnel: [w229 w232 w236 w241 w243 w245 w247 w249 w251 w253 w255 w257 w259 w261 w263 w265 w267 w269 w271 w273 w275 w277 w279 w281 w283 w285 w287 w289 w291 w293 w295 w297 w299 w301 w303 w305 w307 w309 w311 w313 w315 w317 w319 w321 w323 w325 w327 w329 w331 w333 w335 w337 w339 w341 w343 w345 w347 w349 w351 w353 w355 w357 w359 w361 w363 w365 w367 w369 w371 w373 w375 w377 w379 w381 w383 w385 w387 w389 w391 w393 w395 w397 w399 w401 w403 w405 w407 w409 w411 w413 w415 w417 w419 w421 w423 w425 w427 w429 w431 w433 w435 w437 w439 w441 w443] -> w144
          tunnel: w167 -> [w227 w231 w235 w239 _ _ _ _ _ _ _ _ _ _ _ _ _ _ _ _ _ _ _ _ _ _ _ _ _ _ _ _ _ _ _ _ _ _ _ _ _ _ _ _ _ _ _ _ _ _ _ _ _ _ _ _ _ _ _ _ _ _ _ _ _ _ _ _ _ _ _ _ _ _ _ _ _ _ _ _ _ _ _ _ _ _ _ _ _ _ _ _ _ _ _ _ _ _ _ _ _ _ _ _ _]
          frame "DOWN" {
            n126 = Add(x=w230, y=w227) -> (x+y=w229:sgl)
          }
          frame "LEFT" {
            n127 = Subtract(x=w234, y=w231) -> (x-y=w233:sgl)
          }
          frame "RIGHT" {
            n128 = Add(x=w238, y=w235) -> (x+y=w237:sgl)
          }
          frame "UP" {
            n129 = Subtract(x=w242, y=w239) -> (x-y=w241:sgl)
          }
          frame "ENTER (num pad)" {
          }
          frame "' (quote)" {
          }
          frame "END" {
          }
          frame "EQUALS" {
          }
          frame "ESCAPE" {
          }
          frame "GRAVE (`)" {
          }
          frame "HOME" {
          }
          frame "INSERT" {
          }
          frame "LBRACKET" {
          }
          frame "LCONTROL" {
          }
          frame "L ALT" {
          }
          frame "LSHIFT" {
          }
          frame "LWIN" {
          }
          frame "MINUS" {
          }
          frame "MULTIPLY" {
          }
          frame "NEXT" {
          }
          frame "NUMLOCK" {
          }
          frame "NUMPAD_0" {
          }
          frame "NUMPAD_1" {
          }
          frame "NUMPAD_2" {
          }
          frame "NUMPAD_3" {
          }
          frame "NUMPAD_4" {
          }
          frame "NUMPAD_5" {
          }
          frame "NUMPAD_6" {
          }
          frame "NUMPAD_7" {
          }
          frame "NUMPAD_8" {
          }
          frame "NUMPAD_9" {
          }
          frame "PAUSE" {
          }
          frame "PERIOD" {
          }
          frame "PRIOR (PG UP)" {
          }
          frame "RBRACKET" {
          }
          frame "RCONTROL" {
          }
          frame "RETURN" {
          }
          frame "R ALT" {
          }
          frame "RSHIFT" {
          }
          frame "RWIN" {
          }
          frame "SCROLL" {
          }
          frame "SEMICOLON" {
          }
          frame "SLASH" {
          }
          frame "SPACE" {
          }
          frame "SUBTRACT" {
          }
          frame "TAB" {
          }
          frame "DIVIDE" {
          }
          frame "DELETE" {
          }
          frame "DECIMAL" {
          }
          frame "COMMA" {
          }
          frame "CAPITAL" {
          }
          frame "BACKSLASH" {
          }
          frame "BACK" {
          }
          frame "ADD" {
          }
          frame "F15" {
          }
          frame "F14" {
          }
          frame "F13" {
          }
          frame "F12" {
          }
          frame "F11" {
          }
          frame "F10" {
          }
          frame "F9" {
          }
          frame "F8" {
          }
          frame "F7" {
          }
          frame "F6" {
          }
          frame "F5" {
          }
          frame "F4" {
          }
          frame "F3" {
          }
          frame "F2" {
          }
          frame "F1" {
          }
          frame "Z" {
          }
          frame "Y" {
          }
          frame "X" {
          }
          frame "W" {
          }
          frame "V" {
          }
          frame "U" {
          }
          frame "T" {
          }
          frame "S" {
          }
          frame "R" {
          }
          frame "Q" {
          }
          frame "P" {
          }
          frame "O" {
          }
          frame "N" {
          }
          frame "M" {
          }
          frame "L" {
          }
          frame "K" {
          }
          frame "J" {
          }
          frame "I" {
          }
          frame "H" {
          }
          frame "G" {
          }
          frame "F" {
          }
          frame "E" {
          }
          frame "D" {
          }
          frame "C" {
          }
          frame "B" {
          }
          frame "A" {
          }
          frame "9" {
          }
          frame "8" {
          }
          frame "7" {
          }
          frame "6" {
          }
          frame "5" {
          }
          frame "4" {
          }
          frame "3" {
          }
          frame "2" {
          }
          frame "1" {
          }
          frame "0" {
          }
        }
        n130 = To Long Integer(number=w110) -> (32bit integer=w109:i32)
        n131 = To Long Integer(number=w106) -> (32bit integer=w105:i32)
        n132 = To Long Integer(number=w108) -> (32bit integer=w107:i32)
        n133 = To Long Integer(number=w112) -> (32bit integer=w111:i32)
        n134 = Divide(x=w92, y=w94) -> (x/y=w93:dbl)
        n135 = property on="Previous File" class="Bool (strict)"(error in=w179, "Value"=w172) -> (error out=w178:errorcluster)  [unwired: 1 in, 1 out]
        n136 = Divide(x=sgl 20.0, y=w168) -> (x/y=w166:sgl)
        n137 = Bundle(w143, w144) -> (w115:cluster{sgl, sgl})  [unwired: 1 in]
        n138 = Bundle(w109, w111, w107, w105, 0.0) -> (w113:cluster{i32, i32, i32, i32, dbl})  [unwired: 1 in]
        n139 = Multiply(x=w93, y=100) -> (x*y=→"Progress":dbl)
        n140 = To Unsigned Long Integer(number=w115) -> (unsigned 32bit integer=w114:cluster{u32, u32})
        n141 = property on="Save" class="Bool (strict)"(error in=w178, "Value"=w172) -> (error out=w177:errorcluster)  [unwired: 1 in, 1 out]
        n142 = property on="Export" class="Bool (strict)"("Value"=w172) -> ()  [unwired: 2 in, 2 out]
        n143 = call "IMAQ Convert Rectangle to ROI (Polygon)"("Rectangle"=w113) -> ("ROI Descriptor"=w149:T15)  [unwired: 7 in, 2 out]
        n144 = property on="Save Next" class="Bool (strict)"(error in=w177, "Value"=w172) -> (error out=w176:errorcluster)  [unwired: 1 in, 1 out]
        n145 = property on="Discard" class="Bool (strict)"(error in=w176, "Value"=w172) -> (error out=w175:errorcluster)  [unwired: 1 in, 1 out]
        n146 = property on="Save Lines" class="Bool (strict)"(error in=w175, "Value"=w172) -> ()  [unwired: 1 in, 2 out]
        n147 = property on="Image Preview" class="ImageControl"("ROI"=w149) -> ()  [unwired: 2 in, 2 out]
        n148 = property on="Close" class="Bool (strict)"("Value"=w172) -> ()  [unwired: 2 in, 2 out]
        n149 = Bundle("Application Font", w166, w162, w162, w162, w162, w162, TRUE, w164) -> (w161:T16)  [unwired: 1 in]
        n150 = property on="Image Out" class="ImageControl"("Image Center Position"=w114) -> ()  [unwired: 2 in, 2 out]
        n151 = property on="Disable Flag" class="Bool (strict)"("Value"=w172) -> ()  [unwired: 2 in, 2 out]
        n152 = Bundle(w164, w161, w164, w164) -> (w126:T17)  [unwired: 1 in]
        n153 = Cluster To Array(cluster=w171) -> (array=w189:bool[])
        n154 = local read "Image Out"() -> (w125:T8)
        n155 = property on="Image Out" class="ImageControl"() -> ("ROI"=w128:T18)  [unwired: 2 in, 2 out]
        n156 = Unbundle By Name(w128) -> ("Contours"=w129:T19)
        n157 = call "IMAQ Clear Overlay"("Image"=w125) -> ("Image Out"=w142:T8)  [unwired: 9 in, 1 out]
        n158 = Initialize Array(0) -> (w131:i32[])  [unwired: 1 in]
        n159 = Array Size(array=w129) -> (size(s)=w130:i32)
        n160 = call "Next State.vi"("Buttons []"=w189, "States []"=w190) -> ("Save Next?"=→"Save Next?":bool, "Enum"=w182:T2)
        n161 = event shown="[8] \"Transfer File\": Value Change" {
          selector: _ -> [_ _ _ _ _ _ _ _ _ _ _ _ _ _ _]
          dyn-events: _ -> [_ _ _ _ _ _ _ _ _ _ _ _ _ _ _]
          timeout: 5 -> [_ _ _ _ _ _ _ _ _ _ _ _ _ _ _]
          tunnel: w182 -> [w446 _ _ _ _ _ _ _ _ _ _ _ _ _ _]
          tunnel: [w446 MegaAwesome_States."Re-Calculated Values" MegaAwesome_States."Calculated Values" MegaAwesome_States."Re-Calculated Values" MegaAwesome_States."Re-Calculated Values" MegaAwesome_States."Re-Calculated Values" MegaAwesome_States."Re-Calculated Values" MegaAwesome_States."Read Data" MegaAwesome_States."Read Data" MegaAwesome_States."No Event" MegaAwesome_States."No Event" MegaAwesome_States."No Event" MegaAwesome_States."No Event" MegaAwesome_States."No Event" MegaAwesome_States."No Event"] -> w181
          tunnel: w92 -> [w445 w447 w449 w451 w476 w504 w528 _ w557 w559 w572 w574 w578 w582 w586]
          tunnel: [w445 w447 w449 w451 w476 w504 w528 w547 w557 w559 w572 w574 w578 w582 w586] -> w174
          tunnel: w173 -> [_ _ _ _ _ _ _ w546 _ _ _ _ _ _ _]
          tunnel: w171 -> [_ _ _ _ _ _ _ _ _ _ _ _ _ _ _]
          event Timeout {
            n162 = event-data() -> ()  [unwired: 1 in, 2 out]
          }
          event "New: Dielectric", "New: Width", "New: Length", "New: Temp": Value Change {
            n163 = event-data() -> ()  [unwired: 1 in, 5 out]
          }
          event "Num Pts Log", "Transport Style Controls", "Num Pts": Value Change {
            n164 = event-data() -> ()  [unwired: 1 in, 5 out]
          }
          event "Sat-Trans Slider": Value Change {
            n165 = event-data() -> ()  [unwired: 1 in, 5 out]
            n166 = local read "Sqrt-Sat"() -> (w475:cluster{dbl[], dbl[]}[])
            n167 = Decimate 1D Array(w475) -> (w459:cluster{dbl[], dbl[]}[], w460:cluster{dbl[], dbl[]}[])
            n168 = local read "Slider Min"() -> (w456:dbl)
            n169 = local read "Sat-Trans Slider"() -> (w454:dbl)
            n170 = Array To Cluster(array=w459) -> (cluster=w474:T20)
            n171 = local read "New: Dielectric"() -> (w469:dbl)
            n172 = local read "Num Pts"() -> (w452:i32)
            n173 = local read "New: Width"() -> (w471:dbl)
            n174 = local read "New: Length"() -> (w470:dbl)
            n175 = Unbundle(w474) -> ("[0]"=w473:cluster{dbl[], dbl[]})  [unwired: 8 out]
            n176 = Absolute Value(x=w456) -> (abs(x)=w455:dbl)
            n177 = Unbundle(w473) -> (w457:dbl[], w472:dbl[])
            n178 = Add(x=w454, y=w455) -> (x+y=w453:dbl)
            n179 = Array Subset(array=w457, index=w453, length=w452) -> (w467:dbl[])
            n180 = local write "Sat Vg Array-Used"(w467) -> ()
            n181 = Array Subset(array=w472, index=w453, length=w452) -> (w468:dbl[])
            n182 = call "Mobility-Vt-Used Pts_Saturation.vi"("Width"=w471, "Length"=w470, "Dielectric (d)"=w469, "Sat Id Used"=w468, "Vg Used"=w467) -> ("Vt"=w463:dbl, "Mobility"=w464:dbl)  [unwired: 4 in, 1 out]
            n183 = local write "Index-Sat"(w453) -> ()
            n184 = local write "Sat Id-Used"(w468) -> ()
            n185 = Bundle(w467, w468) -> (w461:cluster{dbl[], dbl[]})  [unwired: 1 in]
            n186 = local read "Re-Calculated Values Cluster"() -> (w466:T9)
            n187 = Bundle By Name(cluster=w466, "Mobility-Sat"=w464, "Vt-Sat"=w463) -> (w465:T9)
            n188 = local write "Re-Calculated Values Cluster"(w465) -> ()
            n189 = Build Array (concatenate)(w459, w460, w461) -> (w458:cluster{dbl[], dbl[]}[])
            n190 = local write "Sqrt-Sat"(w458) -> ()
          }
          event "Lin-Trans Slider": Value Change {
            n191 = event-data() -> ()  [unwired: 1 in, 5 out]
            n192 = local read "Sqrt-Lin"() -> (w500:cluster{dbl[], dbl[]}[])
            n193 = Decimate 1D Array(w500) -> (w485:cluster{dbl[], dbl[]}[], w486:cluster{dbl[], dbl[]}[])
            n194 = local read "Slider Min"() -> (w482:dbl)
            n195 = Array To Cluster(array=w485) -> (cluster=w499:T20)
            n196 = local read "Lin-Trans Slider"() -> (w480:dbl)
            n197 = local read "New: Dielectric"() -> (w493:dbl)
            n198 = local read "Num Pts"() -> (w496:i32)
            n199 = local read "New: Width"() -> (w495:dbl)
            n200 = local read "New: Length"() -> (w494:dbl)
            n201 = local read "Lin Vd"() -> (w477:dbl)
            n202 = Unbundle(w499) -> ("[0]"=w498:cluster{dbl[], dbl[]})  [unwired: 8 out]
            n203 = Absolute Value(x=w482) -> (abs(x)=w481:dbl)
            n204 = Unbundle(w498) -> (w483:dbl[], w497:dbl[])
            n205 = Add(x=w480, y=w481) -> (x+y=w479:dbl)
            n206 = Array Subset(array=w483, index=w479, length=w496) -> (w491:dbl[])
            n207 = local write "Lin-Vg Array-Used"(w491) -> ()
            n208 = Array Subset(array=w497, index=w479, length=w496) -> (w492:dbl[])
            n209 = call "Mobility-Vt-Used Pts_Linear.vi"("Width"=w495, "Length"=w494, "Vd"=w477, "Dielectric (d)"=w493, "Id Used"=w492, "Vg Used"=w491) -> ("Mobility"=w488:dbl)  [unwired: 3 in, 2 out]
            n210 = local write "Index-Lin"(w479) -> ()
            n211 = local write "Lin Id-Used"(w492) -> ()
            n212 = Bundle(w491, w492) -> (w487:cluster{dbl[], dbl[]})  [unwired: 1 in]
            n213 = local read "Re-Calculated Values Cluster"() -> (w490:T9)
            n214 = Bundle By Name(cluster=w490, "Moblitity-Lin"=w488) -> (w489:T9)
            n215 = local write "Re-Calculated Values Cluster"(w489) -> ()
            n216 = Build Array (concatenate)(w485, w486, w487) -> (w484:cluster{dbl[], dbl[]}[])
            n217 = local write "Sqrt-Lin"(w484) -> ()
          }
          event "Sat-Log Slider": Value Change {
            n218 = event-data() -> ()  [unwired: 1 in, 5 out]
            n219 = local read "Sat-Log"() -> (w507:cluster{dbl[], dbl[]}[])
            n220 = Decimate 1D Array(w507) -> (w514:cluster{dbl[], dbl[]}[], w515:cluster{dbl[], dbl[]}[])
            n221 = local read "Slider Min"() -> (w511:dbl)
            n222 = Array To Cluster(array=w514) -> (cluster=w524:T20)
            n223 = property on="Sat-Log" class="XYGraph (strict)"("Active Plot"=u32 2, "Plot.Fill/Pt. Color"=u32 6618880, "Plot.Point Style"=u8 11) -> ()  [unwired: 2 in, 2 out]
            n224 = local read "Num Pts Log"() -> (w521:i32)
            n225 = local read "Sat-Log Slider"() -> (w509:dbl)
            n226 = Unbundle(w524) -> ("[0]"=w523:cluster{dbl[], dbl[]})  [unwired: 8 out]
            n227 = Absolute Value(x=w511) -> (abs(x)=w510:dbl)
            n228 = Unbundle(w523) -> (w512:dbl[], w522:dbl[])
            n229 = Add(x=w509, y=w510) -> (x+y=w506:dbl)
            n230 = Array Subset(array=w512, index=w506, length=w521) -> (w519:dbl[])
            n231 = Array Subset(array=w522, index=w506, length=w521) -> (w520:dbl[])
            n232 = local write "Vg Array-Log-Used"(w519) -> ()
            n233 = local write "IndexLog-Sat"(w506) -> ()
            n234 = Bundle(w519, w520) -> (w505:cluster{dbl[], dbl[]})  [unwired: 1 in]
            n235 = call "STS-Used.vi"("Id Used"=w520, "Vg-Used"=w519) -> ("STS"=w516:dbl)  [unwired: 9 in]
            n236 = local write "Sat Id-Log-Used"(w520) -> ()
            n237 = local read "Re-Calculated Values Cluster"() -> (w518:T9)
            n238 = Bundle By Name(cluster=w518, "STS"=w516) -> (w517:T9)
            n239 = local write "Re-Calculated Values Cluster"(w517) -> ()
            n240 = Build Array (concatenate)(w514, w515, w505) -> (w513:cluster{dbl[], dbl[]}[])
            n241 = local write "Sat-Log"(w513) -> ()
          }
          event "Lin-Log Slider": Value Change {
            n242 = event-data() -> ()  [unwired: 1 in, 5 out]
            n243 = local read "Lin-Log"() -> (w532:cluster{dbl[], dbl[]}[])
            n244 = Decimate 1D Array(w532) -> (w538:cluster{dbl[], dbl[]}[], w539:cluster{dbl[], dbl[]}[])
            n245 = local read "Slider Min"() -> (w535:dbl)
            n246 = Array To Cluster(array=w538) -> (cluster=w545:T20)
            n247 = local read "Num Pts Log"() -> (w542:i32)
            n248 = property on="Lin-Log" class="XYGraph (strict)"("Active Plot"=u32 2, "Plot.Fill/Pt. Color"=u32 6618880, "Plot.Point Style"=u8 11) -> ()  [unwired: 2 in, 2 out]
            n249 = local read "Lin-Log Slider"() -> (w533:dbl)
            n250 = Unbundle(w545) -> ("[0]"=w544:cluster{dbl[], dbl[]})  [unwired: 8 out]
            n251 = Absolute Value(x=w535) -> (abs(x)=w534:dbl)
            n252 = Unbundle(w544) -> (w536:dbl[], w543:dbl[])
            n253 = Add(x=w533, y=w534) -> (x+y=w531:dbl)
            n254 = Array Subset(array=w536, index=w531, length=w542) -> (w540:dbl[])
            n255 = local write "Lin-Vg Array-Log Used"(w540) -> ()
            n256 = Array Subset(array=w543, index=w531, length=w542) -> (w541:dbl[])
            n257 = local write "IndexLog-Sat"(w531) -> ()
            n258 = Bundle(w540, w541) -> (w530:cluster{dbl[], dbl[]})  [unwired: 1 in]
            n259 = local write "Lin Id-Log Used"(w541) -> ()
            n260 = Build Array (concatenate)(w538, w539, w530) -> (w537:cluster{dbl[], dbl[]}[])
            n261 = local write "Lin-Log"(w537) -> ()
          }
          event "Index Array": Value Change {
            n262 = event-data() -> ()  [unwired: 1 in, 5 out]
            n263 = Strip Path(path=w546) -> (stripped path=w552:path)  [unwired: 1 out]
            n264 = local write "Transfer Folder"(w552) -> ()
            n265 = List Folder(path=w552) -> (filenames=w548:string[])  [unwired: 3 in, 3 out]
            n266 = local read "Index Array"() -> (w547:i32)
            n267 = Path To String(path=w552) -> (string=w553:string)
            n268 = Index Array(array=w548, index=w547) -> (element=w554:string)
            n269 = Concatenate Strings(w553, "\\", w554) -> (w550:string)
            n270 = String To Path(string=w550) -> (path=w549:path)
            n271 = local write "Transfer File"(w549) -> ()
          }
          event "Transfer File": Value Change {
            w556 = path ""
            n272 = event-data() -> ()  [unwired: 1 in, 5 out]
            n273 = local write "Transport\nFolder"(w556) -> ()
            n274 = local write "Image Folder"(w556) -> ()
          }
          event "Remove Button": Mouse Down {
            w561 = 0
            n275 = event-data() -> ()  [unwired: 1 in, 5 out]
            n276 = property on="Image Out" class="ImageControl"() -> ("ROI"=w571:T18)  [unwired: 2 in, 2 out]
            n277 = Unbundle(w571) -> ("Global Rectangle"=w562:i32[], "Contours"=w564:T19)
            n278 = Reverse 1D Array(array=w562) -> (reversed array=w563:i32[])
            n279 = Reverse 1D Array(array=w564) -> (reversed array=w565:T19)
            n280 = Delete From Array(array=w563, index=w561) -> (array with subset deleted=w566:i32[])  [unwired: 1 in, 1 out]
            n281 = Delete From Array(array=w565, index=w561) -> (array with subset deleted=w567:T19)  [unwired: 1 in, 1 out]
            n282 = Reverse 1D Array(array=w566) -> (reversed array=w568:i32[])
            n283 = Reverse 1D Array(array=w567) -> (reversed array=w569:T19)
            n284 = Bundle(w568, w569) -> (w570:T21)  [unwired: 1 in]
            n285 = property on="Image Out" class="ImageControl"("ROI"=w570) -> ()  [unwired: 2 in, 2 out]
          }
          event "Undo Button": Mouse Down {
            n286 = event-data() -> ()  [unwired: 1 in, 5 out]
            n287 = invoke on="Image Out" class="ImageControl" method="Clear ROI"() -> ()  [unwired: 3 in, 3 out]
          }
          event "Image Folder": Value Change {
            n288 = event-data() -> ()  [unwired: 1 in, 5 out]
            n289 = local read "Image File"() -> (w576:path)
            n290 = call "Vision Acquisition"("Image Path"=w576) -> ("Image Out"=w577:T8)  [unwired: 25 in, 1 out]
            n291 = local write "Image Preview"(w577) -> ()
            n292 = local write "Image Out"(w577) -> ()
          }
          event "Zoom": Value Change {
            n293 = event-data() -> ()  [unwired: 1 in, 5 out]
            n294 = local read "Zoom"() -> (w581:i32)
            n295 = Bundle("Zoom"=w581, "Zoom"=w581) -> (w580:cluster{"Zoom":i32, "Zoom":i32})  [unwired: 1 in]
            n296 = property on="Image Out" class="ImageControl"("ZoomInteger"=w580) -> ()  [unwired: 2 in, 2 out]
          }
          event "Image Out": Mouse Enter {
            n297 = event-data() -> ()  [unwired: 1 in, 3 out]
            n298 = call "Simulate_Keyboard.vi"("Action"=u32 0, "Virtual Key"=u8 162) -> ()  [unwired: 7 in, 1 out]
          }
          event "Image Out": Mouse Leave {
            n299 = event-data() -> ()  [unwired: 1 in, 3 out]
            n300 = flat-sequence {
              frame #0 {
                n301 = Wait (ms)(milliseconds to wait=u32 10) -> ()  [unwired: 1 out]
              }
              frame #1 {
                n302 = call "Simulate_Keyboard.vi"("Action"=u32 2, "Virtual Key"=u8 162) -> ()  [unwired: 7 in, 1 out]
              }
            }
          }
        }
        n303 = Build Array(0.505025, 0.252522, 0.127742, 0.050345, 0.031129) -> (w138:dbl[])
        n304 = Array Subset(array=w138, index="Magnification", length=1) -> (w140:dbl[])
        n305 = To Double Precision Float(number=w140) -> (double precision float=w141:dbl[])
        n306 = for {
          N: w130 -> [_]
          shift-right: [w217] -> _
          shift-left: w129 -> [w217]
          shift-right: [w194] -> w117
          shift-left: w131 -> [w215]
          tunnel: w141 -> [w214]
          shift-right: [w211] -> _
          shift-left: w142 -> [w213]
          tunnel: w126 -> [w207]
          i -> [w210]
          n307 = Index Array(array=w217, index=w210) -> (element=w226:T22)
          n308 = Unbundle(w226) -> ("Points"=w225:i32[])  [unwired: 2 out]
          n309 = Array To Cluster(array=w225) -> (cluster=w224:T23)
          n310 = Unbundle(w224) -> ("Points[0]"=w206:i32, "Points[1]"=w193:i32, "Points[2]"=w216:i32, "Points[3]"=w222:i32)  [unwired: 5 out]
          n311 = Add(x=w206, y=10) -> (x+y=w204:i32)
          n312 = Subtract(x=w193, y=w222) -> (x-y=w221:i32)
          n313 = Subtract(x=w206, y=w216) -> (x-y=w223:i32)
          n314 = Square(x=w221) -> (x^2=w219:i32)
          n315 = Square(x=w223) -> (x^2=w220:i32)
          n316 = To Double Precision Float(number=w193) -> (double precision float=w192:dbl)
          n317 = Add(x=w220, y=w219) -> (x+y=w218:i32)
          n318 = Square Root(x=w218) -> (sqrt(x)=w198:dbl)
          n319 = Multiply(x=w198, y=0.5) -> (x*y=w201:dbl)
          n320 = Multiply(x=w198, y=w214) -> (x*y=w197:dbl[])
          n321 = Index Array(array=w197) -> (element=w209:dbl)  [unwired: 1 in]
          n322 = Number To Fractional String(number=w209, precision (6)=0) -> (F-format string=w208:string)  [unwired: 2 in]
          n323 = Build Array (concatenate)(w215, w197) -> (w195:dbl[])
          n324 = Add(x=w201, y=w192) -> (x+y=w203:dbl)
          n325 = Bundle(w204, w203) -> (w212:cluster{i32, dbl})  [unwired: 1 in]
          n326 = call "IMAQ Overlay Text"("BG Color (Transparent)"=u32 0, "Text Color (black)"=u32 16448250, "Font, Size & Style"=w207, "String"=w208, "Origin"=w212, "Image"=w213) -> ("Image Out"=w211:T8)  [unwired: 4 in, 1 out]
          n327 = To Long Integer(number=w195) -> (32bit integer=w194:i32[])
        }
        "Distances" <- w117
        n328 = Add Array Elements(numeric array=w117) -> (sum=w127:i32)
        n329 = local write "Total Width"(w127) -> ()
      }
      frame "Read Data" {
        n330 = call "IMAQ Dispose"("All Images? (No)"=TRUE) -> ()  [unwired: 5 in, 1 out]
        n331 = case shown="True" "Disable Flag" {
          tunnel: w637 -> [_ w662]
          tunnel: [w658 w659] -> w636
          tunnel: w634 -> [w658 _]
          frame False {
          }
          frame True {
            n332 = local read "Transfer Folder"() -> (w661:path)
            n333 = List Folder(path=w661) -> (filenames=w663:string[])  [unwired: 3 in, 3 out]
            n334 = Index Array(array=w663, index=w662) -> (element=w660:string)
            n335 = Build Path(base path=w661, name or relative path=w660) -> (appended path=w659:path)
            n336 = local write "Transfer File"(w659) -> ()
          }
        }
        n337 = call "Recorded Values.vi"("Path"=w636) -> ("Recorded Char"=→"Recorded Values Cluster":T9, "Recorded Prop"=w649:T1, "Fabrication Prop"=w647:T4)  [unwired: 8 in]
        n338 = Strip Path(path=w636) -> (stripped path=w646:path, name=w645:string)
        n339 = local write "Fabrication Prop"(w647) -> ()
        n340 = local write "Recorded Prop"(w649) -> ()
        n341 = Unbundle By Name(w649) -> ("Date Recorded"=→"Date Recorded":string, "Index"=w648:string, "Length"=w642:dbl, "Width"=w641:dbl)  [unwired: 1 out]
        n342 = Unbundle By Name(w649) -> ("Sample Temp"=w651:dbl)
        n343 = Unbundle By Name(w647) -> ("Dielectric (nm)"=w643:dbl, "Comments"=w644:string, "Date Created"=→"Date Created":string)
        n344 = List Folder(path=w646) -> (filenames=w640:string[])  [unwired: 3 in, 3 out]
        n345 = local write "Rec: Dielectric (d)"(w643) -> ()
        n346 = local write "Index"(w648) -> ()
        n347 = local write "Rec: Length"(w642) -> ()
        n348 = local write "Rec: Width"(w641) -> ()
        n349 = Equal To 0?(x=w651) -> (x = 0?=w654:bool)
        n350 = Number To Decimal String(number=w651) -> (decimal integer string=w655:string)  [unwired: 1 in]
        n351 = local write "Comments:"(w644) -> ()
        n352 = Search 1D Array(1D array=w640, element=w645) -> (index of element=w639:i32)  [unwired: 1 in]
        n353 = Equal?(x="", y=w655) -> (x = y?=w653:bool)
        n354 = Index Array(array=w640, index=w639) -> (element=→"Data Name:":string)
        n355 = local write "New: Width"(w641) -> ()
        n356 = local write "New: Length"(w642) -> ()
        n357 = local write "Index Array"(w639) -> ()
        n358 = Or(x=w654, y=w653) -> (x .or. y?=w652:bool)
        n359 = local write "New: Dielectric"(w643) -> ()
        n360 = case shown="True" w652 {
          tunnel: [w664 w665] -> w633
          tunnel: w651 -> [w664 _]
          frame False {
          }
          frame True {
            n361 = local read "Room Temp"() -> (w665:dbl)
          }
        }
        n362 = local write "New: Temp"(w633) -> ()
        n363 = Bundle By Name(cluster=w649, "Sample Temp"=w633) -> (w650:T1)
        n364 = local write "Rec: Temp"(w633) -> ()
        n365 = local write "Recorded Prop"(w650) -> ()
      }
      frame "Calculated Values" {
        n366 = local read "Image Center X"() -> (w667:i32)
        n367 = call "Image from TRF Display.vi"("Image Center X"=w667, "No Image File"=w712, "Image Folder"=w713, "Transfer File"=w682) -> ("Image Preview"=w674:T8, "Image Out"=w675:T8, "Image File"=w676:path, "Image Name"=→"Image Name":string, "ROI File"=w671:path)  [unwired: 3 in]
        n368 = invoke on="Image Out" class="ImageControl" method="Clear ROI"() -> ()  [unwired: 3 in, 3 out]
        n369 = local write "Image File"(w676) -> ()
        n370 = local write "Image Out"(w675) -> ()
        n371 = local write "Image Preview"(w674) -> ()
        n372 = call <vilib>:"Check if File or Folder Exists.vi"("path"=w671) -> ("file or folder exists?"=w672:bool, "dup path"=w673:path)  [unwired: 8 in, 1 out]
        n373 = case shown="True" w672 {
          tunnel: w673 -> [_ w733]
          frame False {
          }
          frame True {
            n374 = Read from Text File(file (use dialog)=w733) -> (text=w737:string)  [unwired: 3 in, 3 out]
            n375 = property on="Image Out" class="ImageControl"() -> ("ROI"=w734:T18)  [unwired: 2 in, 2 out]
            n376 = Unflatten From String(type=w734, binary string=w737) -> (value=w735:T18, error out=w736:errorcluster)  [unwired: 3 in, 1 out]
            n377 = property on="Image Out" class="ImageControl"(error in=w736, "ROI"=w735) -> ()  [unwired: 1 in, 2 out]
          }
        }
        n378 = call "TRF to TSP Plot_09_21_12a_JW.vi"("Transport Graph Properties"="Transport Style Controls", "No Transport File"=w677, "Transport Folder"=w678, "Transfer File"=w682) -> ("Transport"=w683:cluster{ext[], ext[]}[], "Transport File"=→"Transport\nFile":path, "Transport Name"=→"Transport Name:":string)  [unwired: 5 in]
        "Transport" <- w683
        n379 = Array Size(array=w683) -> (size(s)=w681:i32)
        n380 = local read "Image Center X"() -> (w668:i32)
        n381 = for {
          N: w681 -> [_]
          tunnel: "Transport Style Controls" -> [w741]
          i -> [w740]
          n382 = Unbundle By Name(w741) -> ("Transport Line Size"=w738:u16, "Transport Line Color"=w739:u32)
          n383 = property on="Transport" class="XYGraph (strict)"("Active Plot"=w740, "Plot.Plot Color"=w739, "Plot.Line Width"=w738) -> ()  [unwired: 2 in, 2 out]
        }
        n384 = local read "Recorded Prop"() -> (w715:T1)
        n385 = local read "Fabrication Prop"() -> (w722:T4)
        n386 = Bundle("Image Center X"=w668, 0) -> (w670:cluster{"Image Center X":i32, i32})  [unwired: 1 in]
        n387 = property on="Image Out" class="ImageControl"("Image Center Position"=w670) -> ()  [unwired: 2 in, 2 out]
        n388 = local read "Calculated Values Cluster"() -> (w732:T9)
        n389 = call "Mobility-Vt Calculator-File.vi"("NumPts"=w717, "Path"=w682) -> ("Used Points"=w710:T24, "Graph Cluster"=w700:T25, "Lin Vd"=w685:dbl, "Output"=w730:T26)  [unwired: 6 in]
        n390 = call "STS Calculator-File.vi"("NumPts"=w716, "Path"=w682) -> ("Used Points"=w705:T27, "XY Graph-Sat"=w689:cluster{dbl[], dbl[]}[], "XY Graph-Lin"=w686:cluster{dbl[], dbl[]}[], "Ouput"=w725:cluster{"STS-Sat":dbl, "STS-Lin":dbl})  [unwired: 6 in]
        n391 = Unbundle By Name(w722) -> ("Dielectric (nm)"=w720:dbl)
        n392 = Unbundle By Name(w715) -> ("Sample Temp"=w714:dbl)
        n393 = Unbundle By Name(w730) -> ("Mobility-Sat"=w729:dbl, "Vt-Sat"=w721:dbl, "Mobility-Lin"=w728:dbl, "Off I-Sat"=w727:dbl, "On/Off I-Sat"=w726:dbl)  [unwired: 1 out]
        n394 = local write "Lin Vd"(w685) -> ()
        n395 = Unbundle By Name(w725) -> ("STS-Sat"=w719:dbl)  [unwired: 1 out]
        n396 = local write "Sat-Log"(w689) -> ()
        n397 = local write "Lin-Log"(w686) -> ()
        n398 = call "Trap Density_VT.vi"("VT"=w721, "Dielectric"=w720) -> ("Trap Density-VT"=w724:dbl)
        n399 = call "Trap Density_STS.vi"("Temp (T) [K]"=w714, "S.T.S. (S)"=w719, "Dielectric"=w720) -> ("Trap Density (N)"=w723:dbl)  [unwired: 8 in]
        n400 = Bundle By Name(cluster=w732, "Mobility-Sat"=w729, "Moblitity-Lin"=w728, "On/Off"=w726, "Off Current"=w727, "Vt-Sat"=w721, "STS"=w719, "Trap Density-VT"=w724, "Trap Density-STS"=w723) -> (w731:T9)
        n401 = Unbundle By Name(w705) -> ("Sat Vg Used"=w704:dbl[], "Sat Log(Id) Used"=w703:dbl[], "Lin Vg Used"=w702:dbl[], "Lin Log(Id) Used"=w701:dbl[], "STS Index-Sat"=w687:dbl, "STS Index-Lin"=w688:dbl)
        n402 = Unbundle By Name(w710) -> ("Sat Vg Used"=w709:dbl[], "Sat Sqrt(Id) Used"=w708:dbl[], "Lin Vg Used"=w707:dbl[], "Lin Sqrt(Id) Used"=w706:dbl[], "Index-Lin"=w696:dbl, "Index-Sat"=w695:dbl)
        n403 = local write "Vg Array-Log-Used"(w704) -> ()
        n404 = local write "Sat Id-Log-Used"(w703) -> ()
        n405 = local write "Lin-Vg Array-Log Used"(w702) -> ()
        n406 = local write "Lin Id-Log Used"(w701) -> ()
        n407 = local write "IndexLog-Sat"(w687) -> ()
        n408 = local write "Index-Lin"(w688) -> ()
        n409 = local write "Calculated Values Cluster"(w731) -> ()
        n410 = local write "Sat Vg Array-Used"(w709) -> ()
        n411 = local write "Sat Id-Used"(w708) -> ()
        n412 = local write "Lin-Vg Array-Used"(w707) -> ()
        n413 = local write "Lin Id-Used"(w706) -> ()
        n414 = local write "Index-Sat"(w695) -> ()
        n415 = local write "Index-Lin"(w696) -> ()
        n416 = local write "Lin-Log Slider"(w688) -> ()
        n417 = local write "Sat-Log Slider"(w687) -> ()
        n418 = local write "Sat-Trans Slider"(w695) -> ()
        n419 = local write "Lin-Trans Slider"(w696) -> ()
        n420 = Unbundle By Name(w700) -> ("Raw Sat"=w694:cluster{dbl[], dbl[]}[], "Sqrt Sat"=w697:cluster{dbl[], dbl[]}[], "Raw Lin"=w699:cluster{dbl[], dbl[]}[], "Sqrt Lin"=w698:cluster{dbl[], dbl[]}[])
        n421 = Index Array(array=w694) -> (element=w693:cluster{dbl[], dbl[]})  [unwired: 1 in]
        n422 = Unbundle(w693) -> (w692:dbl[])  [unwired: 1 out]
        n423 = Array Max & Min(array=w692) -> (max value=w691:dbl, min value=w690:dbl)  [unwired: 2 out]
        n424 = property on="Sat-Trans Slider" class="Slide (strict)"("Scale.Maximum"=w691, "Scale.Minimum"=w690) -> ()  [unwired: 2 in, 2 out]
        n425 = property on="Lin-Trans Slider" class="Slide (strict)"("Scale.Maximum"=w691, "Scale.Minimum"=w690) -> ()  [unwired: 2 in, 2 out]
        n426 = property on="Sat-Log Slider" class="Slide (strict)"("Scale.Maximum"=w691, "Scale.Minimum"=w690) -> ()  [unwired: 2 in, 2 out]
        n427 = property on="Lin-Log Slider" class="Slide (strict)"("Scale.Maximum"=w691, "Scale.Minimum"=w690) -> ()  [unwired: 2 in, 2 out]
        n428 = local write "Slider Max"(w691) -> ()
        n429 = local write "Slider Min"(w690) -> ()
        n430 = local write "Raw- Sat"(w694) -> ()
        n431 = local write "Raw- Lin"(w699) -> ()
        n432 = local write "Sqrt-Sat"(w697) -> ()
        n433 = local write "Sqrt-Lin"(w698) -> ()
      }
      frame "Re-Calculated Values" {
        n434 = local read "Vg Array-Log-Used"() -> (w750:dbl[])
        n435 = local read "Sat Vg Array-Used"() -> (w758:dbl[])
        n436 = local read "Lin-Vg Array-Used"() -> (w764:dbl[])
        n437 = local read "Sat Id-Log-Used"() -> (w749:dbl[])
        n438 = local read "New: Dielectric"() -> (w762:dbl)
        n439 = local read "New: Dielectric"() -> (w747:dbl)
        n440 = local read "New: Length"() -> (w761:dbl)
        n441 = local read "New: Length"() -> (w757:dbl)
        n442 = local read "New: Width"() -> (w760:dbl)
        n443 = local read "New: Width"() -> (w756:dbl)
        n444 = local read "Lin Id-Used"() -> (w763:dbl[])
        n445 = local read "Sat Id-Used"() -> (w755:dbl[])
        n446 = local read "Re-Calculated Values Cluster"() -> (w766:T9)
        n447 = local read "New: Dielectric"() -> (w746:dbl)
        n448 = local read "New: Temp"() -> (w745:dbl)
        n449 = local read "Lin Vd"() -> (w742:dbl)
        n450 = call "Mobility-Vt-Used Pts_Saturation.vi"("Width"=w756, "Length"=w757, "Dielectric (d)"=w747, "Sat Id Used"=w755, "Vg Used"=w758) -> ("Vt"=w753:dbl, "Mobility"=w754:dbl)  [unwired: 4 in, 1 out]
        n451 = call "STS-Used.vi"("Id Used"=w749, "Vg-Used"=w750) -> ("STS"=w748:dbl)  [unwired: 9 in]
        n452 = call "Mobility-Vt-Used Pts_Linear.vi"("Width"=w760, "Length"=w761, "Vd"=w742, "Dielectric (d)"=w762, "Id Used"=w763, "Vg Used"=w764) -> ("Mobility"=w759:dbl)  [unwired: 3 in, 2 out]
        n453 = call "Trap Density_VT.vi"("VT"=w753, "Dielectric"=w747) -> ("Trap Density-VT"=w752:dbl)
        n454 = call "Trap Density_STS.vi"("Temp (T) [K]"=w745, "S.T.S. (S)"=w748, "Dielectric"=w746) -> ("Trap Density (N)"=w744:dbl)  [unwired: 8 in]
        n455 = Bundle By Name(cluster=w766, "Mobility-Sat"=w754, "Moblitity-Lin"=w759, "Vt-Sat"=w753, "STS"=w748, "Trap Density-VT"=w752, "Trap Density-STS"=w744) -> (w765:T9)
        n456 = local write "Re-Calculated Values Cluster"(w765) -> ()
      }
      frame "Next File" {
        n457 = call "IMAQ Dispose"("All Images? (No)"=TRUE) -> ()  [unwired: 5 in, 1 out]
        n458 = Strip Path(path=w783) -> (stripped path=w774:path, name=w781:string)
        n459 = local write "Transfer Folder"(w774) -> ()
        n460 = List Folder(path=w774) -> (filenames=w768:string[])  [unwired: 3 in, 3 out]
        n461 = Array Size(array=w768) -> (size(s)=w780:i32)
        n462 = Search 1D Array(1D array=w768, element=w781) -> (index of element=w778:i32)  [unwired: 1 in]
        n463 = Decrement(x=w780) -> (x-1=w779:i32)
        n464 = Equal?(x=w779, y=w778) -> (x = y?=w777:bool)
        n465 = case shown="True" w777 {
          tunnel: w770 -> [w785 _]
          tunnel: [w784 0] -> w769
          frame False {
            n466 = Increment(x=w785) -> (x+1=w784:i32)
          }
          frame True {
          }
        }
        n467 = Path To String(path=w774) -> (string=w775:string)
        n468 = Index Array(array=w768, index=w769) -> (element=w776:string)
        n469 = Concatenate Strings(w775, "\\", w776) -> (w772:string)
        n470 = String To Path(string=w772) -> (path=w771:path)
        n471 = local write "Transfer File"(w771) -> ()
      }
      frame "Previous File" {
        n472 = call "IMAQ Dispose"("All Images? (No)"=TRUE) -> ()  [unwired: 5 in, 1 out]
        n473 = Strip Path(path=w794) -> (stripped path=w791:path, name=w802:string)
        n474 = local write "Transfer Folder"(w791) -> ()
        n475 = List Folder(path=w791) -> (filenames=w795:string[])  [unwired: 3 in, 3 out]
        n476 = Array Size(array=w795) -> (size(s)=w789:i32)
        n477 = Search 1D Array(1D array=w795, element=w802) -> (index of element=w801:i32)  [unwired: 1 in]
        n478 = Decrement(x=w789) -> (x-1=w788:i32)
        n479 = Equal To 0?(x=w801) -> (x = 0?=w800:bool)
        n480 = case shown="True" w800 {
          tunnel: w793 -> [w805 _]
          tunnel: [w804 w806] -> w792
          tunnel: w788 -> [_ w806]
          frame False {
            n481 = Decrement(x=w805) -> (x-1=w804:i32)
          }
          frame True {
          }
        }
        n482 = Path To String(path=w791) -> (string=w790:string)
        n483 = Index Array(array=w795, index=w792) -> (element=w799:string)
        n484 = Concatenate Strings(w790, "\\", w799) -> (w797:string)
        n485 = String To Path(string=w797) -> (path=w796:path)
        n486 = local write "Transfer File"(w796) -> ()
      }
      frame "Discard File" {
        n487 = Strip Path(path=w821) -> (stripped path=w809:path, name=w812:string)
        n488 = property on="Disable Flag" class="Bool (strict)"("Value"=TRUE) -> ()  [unwired: 2 in, 2 out]
        n489 = List Folder(path=w809) -> (filenames=w811:string[])  [unwired: 3 in, 3 out]
        n490 = Search 1D Array(1D array=w811, element=w812) -> (index of element=w818:i32)  [unwired: 1 in]
        n491 = call "IMAQ Dispose"("All Images? (No)"=TRUE) -> ()  [unwired: 5 in, 1 out]
        n492 = String Subset(string=w812, offset (0)=0, length (rest)=1) -> (substring=w815:string)
        n493 = Equal?(x=w815, y="X") -> (x = y?=w813:bool)
        n494 = case shown="False" w813 {
          tunnel: w809 -> [w830 _]
          tunnel: w821 -> [w826 _]
          tunnel: w812 -> [w825 _]
          tunnel: w818 -> [w824 w834]
          tunnel: [w823 w833] -> w810
          frame False {
            n495 = Increment(x=w824) -> (x+1=w823:i32)
            n496 = Path To String(path=w830) -> (string=w829:string)
            n497 = Concatenate Strings(w829, "\\", "X_", w825) -> (w828:string)
            n498 = String To Path(string=w828) -> (path=w827:path)
            n499 = Move(source path=w826, 10:w827) -> ()  [unwired: 3 in, 3 out]
          }
          frame True {
            n500 = Increment(x=w834) -> (x+1=w833:i32)
          }
        }
        n501 = Index Array(array=w811, index=w810) -> (element=w808:string)
        n502 = Build Path(base path=w809, name or relative path=w808) -> (appended path=w807:path)
        n503 = local write "Transfer File"(w807) -> ()
      }
      frame "Save" {
        n504 = stacked-sequence {
          seq-local: [w849 _] -> [_ w1331]
          seq-local: [w848 _] -> [_ w1329]
          tunnel: w841 -> [w850 w1332]
          frame #0 {
            # "Saves each Re-calculated parameter in sequence"
            n505 = stacked-sequence {
              tunnel: [_ _ _ _ _ _ _ _ _ _ _ _ _ w1299] -> w848
              tunnel: w850 -> [w870 _ _ _ _ _ _ _ _ _ _ _ _ _]
              frame #0 {
                n506 = call-poly <vilib>:"Read From Spreadsheet File.vi"("file path (dialog if empty)"=w870) -> ("all rows"=w869:string[][])  [unwired: 6 in, 4 out]
                n507 = Array Size(array=w869) -> (size(s)=w874:i32[])
                n508 = Array Subset(array=w869, index (row)=0, index (col)=0, length (col)=3) -> (w878:string[][])  [unwired: 1 in]
                n509 = Index Array(array=w874, index=0) -> (element=w872:i32)
                n510 = Reshape Array(w878, w872) -> (w871:string[])
                n511 = Search 1D Array(1D array=w871, element="Dielectric (nm):") -> (index of element=w881:i32)  [unwired: 1 in]
                n512 = Equal?(x=w881, y=-1) -> (x = y?=w880:bool)
                n513 = case shown="False" w880 {
                  tunnel: w869 -> [w888 w892]
                  tunnel: w881 -> [w886 _]
                  tunnel: [w885 w892] -> w879
                  frame False {
                    n514 = local read "Rec: Dielectric (d)"() -> (w890:dbl)
                    n515 = Number To Fractional String(number=w890) -> (F-format string=w887:string)  [unwired: 3 in]
                    n516 = Quotient & Remainder(x=w886, y=3) -> (floor(x/y)=w884:i32)  [unwired: 1 out]
                    n517 = Replace Array Subset(array=w888, new element=w887, index (row)=w884, index (col)=1) -> (w885:string[][])
                  }
                  frame True {
                  }
                }
                n518 = local write "Save Array"(w879) -> ()
              }
              frame #1 {
                n519 = local read "Save Array"() -> (w894:string[][])
                n520 = Array Size(array=w894) -> (size(s)=w897:i32[])
                n521 = Array Subset(array=w894, index (row)=0, index (col)=0, length (col)=3) -> (w901:string[][])  [unwired: 1 in]
                n522 = Index Array(array=w897, index=0) -> (element=w895:i32)
                n523 = Reshape Array(w901, w895) -> (w893:string[])
                n524 = Search 1D Array(1D array=w893, element="Comments:") -> (index of element=w904:i32)  [unwired: 1 in]
                n525 = Equal?(x=w904, y=-1) -> (x = y?=w903:bool)
                n526 = case shown="False" w903 {
                  tunnel: w894 -> [w912 w914]
                  tunnel: w904 -> [w909 _]
                  tunnel: [w911 w914] -> w902
                  frame False {
                    n527 = local read "Comments:"() -> (w910:string)
                    n528 = Quotient & Remainder(x=w909, y=3) -> (floor(x/y)=w907:i32)  [unwired: 1 out]
                    n529 = Replace Array Subset(array=w912, new element=w910, index (row)=w907, index (col)=1) -> (w911:string[][])
                  }
                  frame True {
                  }
                }
                n530 = local write "Save Array"(w902) -> ()
              }
              frame #2 {
                n531 = local read "Save Array"() -> (w916:string[][])
                n532 = Array Size(array=w916) -> (size(s)=w919:i32[])
                n533 = Array Subset(array=w916, index (row)=0, index (col)=0, length (col)=3) -> (w923:string[][])  [unwired: 1 in]
                n534 = Index Array(array=w919, index=0) -> (element=w917:i32)
                n535 = Reshape Array(w923, w917) -> (w915:string[])
                n536 = Search 1D Array(1D array=w915, element="Length (um):") -> (index of element=w926:i32)  [unwired: 1 in]
                n537 = Equal?(x=w926, y=-1) -> (x = y?=w925:bool)
                n538 = case shown="False" w925 {
                  tunnel: w916 -> [w935 w938]
                  tunnel: w926 -> [w934 _]
                  tunnel: [w933 w938] -> w924
                  frame False {
                    n539 = local read "New: Length"() -> (w930:dbl)
                    n540 = Quotient & Remainder(x=w934, y=3) -> (floor(x/y)=w929:i32)  [unwired: 1 out]
                    n541 = Format Value(format string="%#g", value (0)=w930) -> (output string=w931:string)  [unwired: 1 in]
                    n542 = Replace Array Subset(array=w935, new element=w931, index (row)=w929, index (col)=1) -> (w933:string[][])
                  }
                  frame True {
                  }
                }
                n543 = local write "Save Array"(w924) -> ()
              }
              frame #3 {
                n544 = local read "Save Array"() -> (w940:string[][])
                n545 = Array Size(array=w940) -> (size(s)=w945:i32[])
                n546 = Array Subset(array=w940, index (row)=0, index (col)=0, length (col)=3) -> (w941:string[][])  [unwired: 1 in]
                n547 = Index Array(array=w945, index=0) -> (element=w947:i32)
                n548 = Reshape Array(w941, w947) -> (w939:string[])
                n549 = Search 1D Array(1D array=w939, element="Width (um):") -> (index of element=w950:i32)  [unwired: 1 in]
                n550 = Equal?(x=w950, y=-1) -> (x = y?=w949:bool)
                n551 = case shown="False" w949 {
                  tunnel: w950 -> [w959 _]
                  tunnel: w940 -> [w958 w962]
                  tunnel: [w957 w962] -> w948
                  frame False {
                    n552 = local read "New: Width"() -> (w954:dbl)
                    n553 = Quotient & Remainder(x=w959, y=3) -> (floor(x/y)=w953:i32)  [unwired: 1 out]
                    n554 = Format Value(format string="%#g", value (0)=w954) -> (output string=w955:string)  [unwired: 1 in]
                    n555 = Replace Array Subset(array=w958, new element=w955, index (row)=w953, index (col)=1) -> (w957:string[][])
                  }
                  frame True {
                  }
                }
                n556 = local write "Save Array"(w948) -> ()
              }
              frame #4 {
                w972 = "Sample Temp (K):"
                n557 = local read "Save Array"() -> (w964:string[][])
                n558 = Array Size(array=w964) -> (size(s)=w969:i32[])
                n559 = Array Subset(array=w964, index (row)=0, index (col)=0, length (col)=3) -> (w965:string[][])  [unwired: 1 in]
                n560 = Index Array(array=w969, index=0) -> (element=w971:i32)
                n561 = Reshape Array(w965, w971) -> (w963:string[])
                n562 = Search 1D Array(1D array=w963, element=w972) -> (index of element=w975:i32)  [unwired: 1 in]
                n563 = Equal?(x=w975, y=-1) -> (x = y?=w974:bool)
                n564 = case shown="False" w974 {
                  tunnel: w964 -> [w983 w996]
                  tunnel: w975 -> [w982 _]
                  tunnel: [w981 w995] -> w973
                  tunnel: w963 -> [_ w998]
                  tunnel: w972 -> [_ w987]
                  frame False {
                    n565 = local read "New: Temp"() -> (w979:dbl)
                    n566 = Quotient & Remainder(x=w982, y=3) -> (floor(x/y)=w977:i32)  [unwired: 1 out]
                    n567 = Format Value(format string="%#g", value (0)=w979) -> (output string=w978:string)  [unwired: 1 in]
                    n568 = Replace Array Subset(array=w983, new element=w978, index (row)=w977, index (col)=1) -> (w981:string[][])
                  }
                  frame True {
                    n569 = local read "New: Temp"() -> (w989:dbl)
                    n570 = Search 1D Array(1D array=w998, element="Width (um):") -> (index of element=w993:i32)  [unwired: 1 in]
                    n571 = Quotient & Remainder(x=w993, y=3) -> (floor(x/y)=w986:i32)  [unwired: 1 out]
                    n572 = Increment(x=w986) -> (x+1=w992:i32)
                    n573 = Format Value(format string="%#g", value (0)=w989) -> (output string=w988:string)  [unwired: 1 in]
                    n574 = Build Array(w987, w988) -> (w991:string[])
                    n575 = Insert Into Array(array=w996, index (row)=w992, new element=w991) -> (w995:string[][])  [unwired: 1 in]
                  }
                }
                n576 = local write "Save Array"(w973) -> ()
              }
              frame #5 {
                w1008 = "Mobility-Sat (cm^2/Vs):"
                n577 = local read "Save Array"() -> (w1000:string[][])
                n578 = Array Size(array=w1000) -> (size(s)=w1005:i32[])
                n579 = Array Subset(array=w1000, index (row)=0, index (col)=0, length (col)=3) -> (w1001:string[][])  [unwired: 1 in]
                n580 = Index Array(array=w1005, index=0) -> (element=w1007:i32)
                n581 = Reshape Array(w1001, w1007) -> (w999:string[])
                n582 = Search 1D Array(1D array=w999, element=w1008) -> (index of element=w1011:i32)  [unwired: 1 in]
                n583 = Equal?(x=w1011, y=-1) -> (x = y?=w1010:bool)
                n584 = case shown="False" w1010 {
                  tunnel: w1000 -> [w1020 w1030]
                  tunnel: w1011 -> [w1019 _]
                  tunnel: [w1018 w1029] -> w1009
                  tunnel: w999 -> [_ w1027]
                  tunnel: w1008 -> [_ w1026]
                  frame False {
                    n585 = local read "Re-Calculated Values Cluster"() -> (w1015:T9)
                    n586 = Unbundle By Name(w1015) -> ("Mobility-Sat"=w1014:dbl)
                    n587 = Quotient & Remainder(x=w1019, y=3) -> (floor(x/y)=w1013:i32)  [unwired: 1 out]
                    n588 = Format Value(format string="%#g", value (0)=w1014) -> (output string=w1016:string)  [unwired: 1 in]
                    n589 = Replace Array Subset(array=w1020, new element=w1016, index (row)=w1013, index (col)=1) -> (w1018:string[][])
                  }
                  frame True {
                    n590 = local read "Re-Calculated Values Cluster"() -> (w1025:T9)
                    n591 = Unbundle By Name(w1025) -> ("Mobility-Sat"=w1024:dbl)
                    n592 = Search 1D Array(1D array=w1027, element="Mobility (cm^2/Vs):") -> (index of element=w1033:i32)  [unwired: 1 in]
                    n593 = Quotient & Remainder(x=w1033, y=3) -> (floor(x/y)=w1023:i32)  [unwired: 1 out]
                    n594 = Format Value(format string="%#g", value (0)=w1024) -> (output string=w1028:string)  [unwired: 1 in]
                    n595 = Build Array(w1026, w1028) -> (w1032:string[])
                    n596 = Replace Array Subset(array=w1030, new element=w1032, index (row)=w1023) -> (w1029:string[][])  [unwired: 1 in]
                  }
                }
                n597 = local write "Save Array"(w1009) -> ()
              }
              frame #6 {
                w1045 = "Mobility-Lin (cm^2/Vs):"
                n598 = local read "Save Array"() -> (w1036:string[][])
                n599 = Array Size(array=w1036) -> (size(s)=w1042:i32[])
                n600 = Array Subset(array=w1036, index (row)=0, index (col)=0, length (col)=3) -> (w1038:string[][])  [unwired: 1 in]
                n601 = Index Array(array=w1042, index=0) -> (element=w1044:i32)
                n602 = Reshape Array(w1038, w1044) -> (w1037:string[])
                n603 = Search 1D Array(1D array=w1037, element=w1045) -> (index of element=w1048:i32)  [unwired: 1 in]
                n604 = Equal?(x=w1048, y=-1) -> (x = y?=w1047:bool)
                n605 = case shown="True" w1047 {
                  tunnel: w1036 -> [w1057 w1066]
                  tunnel: w1048 -> [w1056 _]
                  tunnel: [w1055 w1065] -> w1046
                  tunnel: w1037 -> [_ w1064]
                  tunnel: w1045 -> [_ w1063]
                  frame False {
                    n606 = local read "Re-Calculated Values Cluster"() -> (w1052:T9)
                    n607 = Unbundle By Name(w1052) -> ("Moblitity-Lin"=w1051:dbl)
                    n608 = Quotient & Remainder(x=w1056, y=3) -> (floor(x/y)=w1050:i32)  [unwired: 1 out]
                    n609 = Format Value(format string="%#g", value (0)=w1051) -> (output string=w1053:string)  [unwired: 1 in]
                    n610 = Replace Array Subset(array=w1057, new element=w1053, index (row)=w1050, index (col)=1) -> (w1055:string[][])
                  }
                  frame True {
                    n611 = local read "Re-Calculated Values Cluster"() -> (w1062:T9)
                    n612 = Unbundle By Name(w1062) -> ("Moblitity-Lin"=w1061:dbl)
                    n613 = Search 1D Array(1D array=w1064, element="Mobility-Sat (cm^2/Vs):") -> (index of element=w1070:i32)  [unwired: 1 in]
                    n614 = Quotient & Remainder(x=w1070, y=3) -> (floor(x/y)=w1060:i32)  [unwired: 1 out]
                    n615 = Format Value(format string="%#g", value (0)=w1061) -> (output string=w1073:string)  [unwired: 1 in]
                    n616 = Build Array(w1063, w1073) -> (w1068:string[])
                    n617 = Increment(x=w1060) -> (x+1=w1069:i32)
                    n618 = Insert Into Array(array=w1066, index (row)=w1069, new element=w1068) -> (w1065:string[][])  [unwired: 1 in]
                  }
                }
                n619 = local write "Save Array"(w1046) -> ()
              }
              frame #7 {
                w1083 = "On/Off I-Sat:"
                n620 = local read "Save Array"() -> (w1074:string[][])
                n621 = Array Size(array=w1074) -> (size(s)=w1080:i32[])
                n622 = Array Subset(array=w1074, index (row)=0, index (col)=0, length (col)=3) -> (w1076:string[][])  [unwired: 1 in]
                n623 = Index Array(array=w1080, index=0) -> (element=w1082:i32)
                n624 = Reshape Array(w1076, w1082) -> (w1075:string[])
                n625 = Search 1D Array(1D array=w1075, element=w1083) -> (index of element=w1086:i32)  [unwired: 1 in]
                n626 = Equal?(x=w1086, y=-1) -> (x = y?=w1085:bool)
                n627 = case shown="True" w1085 {
                  tunnel: w1074 -> [w1095 w1104]
                  tunnel: w1086 -> [w1094 _]
                  tunnel: [w1093 w1105] -> w1084
                  tunnel: w1075 -> [_ w1102]
                  tunnel: w1083 -> [_ w1101]
                  frame False {
                    n628 = local read "Calculated Values Cluster"() -> (w1090:T9)
                    n629 = Quotient & Remainder(x=w1094, y=3) -> (floor(x/y)=w1088:i32)  [unwired: 1 out]
                    n630 = Unbundle By Name(w1090) -> ("On/Off"=w1089:dbl)
                    n631 = Format Value(format string="%#g", value (0)=w1089) -> (output string=w1091:string)  [unwired: 1 in]
                    n632 = Replace Array Subset(array=w1095, new element=w1091, index (row)=w1088, index (col)=1) -> (w1093:string[][])
                  }
                  frame True {
                    n633 = local read "Calculated Values Cluster"() -> (w1100:T9)
                    n634 = Unbundle By Name(w1100) -> ("On/Off"=w1099:dbl)
                    n635 = Search 1D Array(1D array=w1102, element="On/Off Current:") -> (index of element=w1108:i32)  [unwired: 1 in]
                    n636 = Quotient & Remainder(x=w1108, y=3) -> (floor(x/y)=w1098:i32)  [unwired: 1 out]
                    n637 = Format Value(format string="%#g", value (0)=w1099) -> (output string=w1103:string)  [unwired: 1 in]
                    n638 = Build Array(w1101, w1103) -> (w1107:string[])
                    n639 = Replace Array Subset(array=w1104, new element=w1107, index (row)=w1098) -> (w1105:string[][])  [unwired: 1 in]
                  }
                }
                n640 = local write "Save Array"(w1084) -> ()
              }
              frame #8 {
                w1120 = "Off I-Sat (A):"
                n641 = local read "Save Array"() -> (w1111:string[][])
                n642 = Array Size(array=w1111) -> (size(s)=w1117:i32[])
                n643 = Array Subset(array=w1111, index (row)=0, index (col)=0, length (col)=3) -> (w1113:string[][])  [unwired: 1 in]
                n644 = Index Array(array=w1117, index=0) -> (element=w1119:i32)
                n645 = Reshape Array(w1113, w1119) -> (w1112:string[])
                n646 = Search 1D Array(1D array=w1112, element=w1120) -> (index of element=w1123:i32)  [unwired: 1 in]
                n647 = Equal?(x=w1123, y=-1) -> (x = y?=w1122:bool)
                n648 = case shown="True" w1122 {
                  tunnel: w1111 -> [w1132 w1141]
                  tunnel: w1123 -> [w1131 _]
                  tunnel: [w1130 w1140] -> w1121
                  tunnel: w1112 -> [_ w1139]
                  tunnel: w1120 -> [_ w1138]
                  frame False {
                    # "New Data File"
                    n649 = local read "Calculated Values Cluster"() -> (w1127:T9)
                    n650 = Unbundle By Name(w1127) -> ("Off Current"=w1126:dbl)
                    n651 = Quotient & Remainder(x=w1131, y=3) -> (floor(x/y)=w1125:i32)  [unwired: 1 out]
                    n652 = Format Value(format string="%#g", value (0)=w1126) -> (output string=w1128:string)  [unwired: 1 in]
                    n653 = Replace Array Subset(array=w1132, new element=w1128, index (row)=w1125, index (col)=1) -> (w1130:string[][])
                  }
                  frame True {
                    # "Old Data File"
                    n654 = local read "Calculated Values Cluster"() -> (w1137:T9)
                    n655 = Unbundle By Name(w1137) -> ("Off Current"=w1136:dbl)
                    n656 = Search 1D Array(1D array=w1139, element="On/Off I-Sat:") -> (index of element=w1145:i32)  [unwired: 1 in]
                    n657 = Quotient & Remainder(x=w1145, y=3) -> (floor(x/y)=w1135:i32)  [unwired: 1 out]
                    n658 = Format Value(format string="%#g", value (0)=w1136) -> (output string=w1148:string)  [unwired: 1 in]
                    n659 = Build Array(w1138, w1148) -> (w1143:string[])
                    n660 = Increment(x=w1135) -> (x+1=w1144:i32)
                    n661 = Insert Into Array(array=w1141, index (row)=w1144, new element=w1143) -> (w1140:string[][])  [unwired: 1 in]
                  }
                }
                n662 = local write "Save Array"(w1121) -> ()
              }
              frame #9 {
                w1150 = "Vt-Sat (V):"
                n663 = local read "Save Array"() -> (w1151:string[][])
                n664 = Array Size(array=w1151) -> (size(s)=w1156:i32[])
                n665 = Array Subset(array=w1151, index (row)=0, index (col)=0, length (col)=3) -> (w1152:string[][])  [unwired: 1 in]
                n666 = Index Array(array=w1156, index=0) -> (element=w1158:i32)
                n667 = Reshape Array(w1152, w1158) -> (w1149:string[])
                n668 = Search 1D Array(1D array=w1149, element=w1150) -> (index of element=w1161:i32)  [unwired: 1 in]
                n669 = Equal?(x=w1161, y=-1) -> (x = y?=w1160:bool)
                n670 = case shown="True" w1160 {
                  tunnel: w1151 -> [w1169 w1181]
                  tunnel: w1161 -> [w1167 _]
                  tunnel: [w1166 w1180] -> w1159
                  tunnel: w1150 -> [_ w1179]
                  tunnel: w1149 -> [_ w1178]
                  frame False {
                    n671 = local read "Re-Calculated Values Cluster"() -> (w1165:T9)
                    n672 = Unbundle By Name(w1165) -> ("Vt-Sat"=w1164:dbl)
                    n673 = Quotient & Remainder(x=w1167, y=3) -> (floor(x/y)=w1163:i32)  [unwired: 1 out]
                    n674 = Number To Fractional String(number=w1164) -> (F-format string=w1168:string)  [unwired: 3 in]
                    n675 = Replace Array Subset(array=w1169, new element=w1168, index (row)=w1163, index (col)=1) -> (w1166:string[][])
                  }
                  frame True {
                    n676 = local read "Re-Calculated Values Cluster"() -> (w1177:T9)
                    n677 = Unbundle By Name(w1177) -> ("Vt-Sat"=w1176:dbl)
                    n678 = Search 1D Array(1D array=w1178, element="Off I-Sat (A):") -> (index of element=w1174:i32)  [unwired: 1 in]
                    n679 = Add(x=w1174, y=3) -> (x+y=w1172:i32)
                    n680 = Quotient & Remainder(x=w1172, y=3) -> (floor(x/y)=w1175:i32)  [unwired: 1 out]
                    n681 = Format Value(format string="%#g", value (0)=w1176) -> (output string=w1186:string)  [unwired: 1 in]
                    n682 = Build Array(w1179, w1186) -> (w1183:string[])
                    n683 = Replace Array Subset(array=w1181, new element=w1183, index (row)=w1175) -> (w1180:string[][])  [unwired: 1 in]
                  }
                }
                n684 = local write "Save Array"(w1159) -> ()
              }
              frame #10 {
                n685 = disable-structure shown="Disabled" {
                  frame Disabled {
                    n686 = local read "Save Array"() -> (w1187:string[][])
                    n687 = Array Size(array=w1187) -> (size(s)=w1193:i32[])
                    n688 = Array Subset(array=w1187, index (row)=0, index (col)=0, length (col)=3) -> (w1189:string[][])  [unwired: 1 in]
                    n689 = Index Array(array=w1193, index=0) -> (element=w1195:i32)
                    n690 = Reshape Array(w1189, w1195) -> (w1188:string[])
                    n691 = Search 1D Array(1D array=w1188, element="VT-Lin (V):") -> (index of element=w1198:i32)  [unwired: 1 in]
                    n692 = Equal?(x=w1198, y=-1) -> (x = y?=w1197:bool)
                    n693 = case shown="True" w1197 {
                      tunnel: w1187 -> [w1206 w1209]
                      tunnel: w1198 -> [w1205 _]
                      tunnel: [w1204 w1209] -> w1196
                      frame False {
                        n694 = Quotient & Remainder(x=w1205, y=3) -> (floor(x/y)=w1201:i32)  [unwired: 1 out]
                        n695 = Format Value(format string="%#g") -> (output string=w1202:string)  [unwired: 2 in]
                        n696 = Replace Array Subset(array=w1206, new element=w1202, index (row)=w1201, index (col)=1) -> (w1204:string[][])
                      }
                      frame True {
                      }
                    }
                    n697 = local write "Save Array"(w1196) -> ()
                  }
                  frame Enabled {
                  }
                }
              }
              frame #11 {
                w1210 = "STS-Sat (V/decade):"
                n698 = local read "Save Array"() -> (w1212:string[][])
                n699 = Array Size(array=w1212) -> (size(s)=w1217:i32[])
                n700 = Array Subset(array=w1212, index (row)=0, index (col)=0, length (col)=3) -> (w1213:string[][])  [unwired: 1 in]
                n701 = Index Array(array=w1217, index=0) -> (element=w1219:i32)
                n702 = Reshape Array(w1213, w1219) -> (w1211:string[])
                n703 = Search 1D Array(1D array=w1211, element=w1210) -> (index of element=w1222:i32)  [unwired: 1 in]
                n704 = Equal?(x=w1222, y=-1) -> (x = y?=w1221:bool)
                n705 = case shown="True" w1221 {
                  tunnel: w1212 -> [w1231 w1242]
                  tunnel: w1222 -> [w1230 _]
                  tunnel: [w1229 w1243] -> w1220
                  tunnel: w1211 -> [_ w1241]
                  tunnel: w1210 -> [_ w1240]
                  frame False {
                    # "Current Data File"
                    n706 = local read "Re-Calculated Values Cluster"() -> (w1225:T9)
                    n707 = Unbundle By Name(w1225) -> ("STS"=w1226:dbl)
                    n708 = Quotient & Remainder(x=w1230, y=3) -> (floor(x/y)=w1224:i32)  [unwired: 1 out]
                    n709 = Format Value(format string="%#g", value (0)=w1226) -> (output string=w1227:string)  [unwired: 1 in]
                    n710 = Replace Array Subset(array=w1231, new element=w1227, index (row)=w1224, index (col)=1) -> (w1229:string[][])
                  }
                  frame True {
                    # "Old Data File"
                    n711 = local read "Re-Calculated Values Cluster"() -> (w1238:T9)
                    n712 = Unbundle By Name(w1238) -> ("STS"=w1239:dbl)
                    n713 = Search 1D Array(1D array=w1241, element="Vt-Sat (V):") -> (index of element=w1235:i32)  [unwired: 1 in]
                    n714 = Add(x=w1235, y=3) -> (x+y=w1234:i32)
                    n715 = Quotient & Remainder(x=w1234, y=3) -> (floor(x/y)=w1237:i32)  [unwired: 1 out]
                    n716 = Format Value(format string="%#g", value (0)=w1239) -> (output string=w1248:string)  [unwired: 1 in]
                    n717 = Build Array(w1240, w1248) -> (w1245:string[])
                    n718 = Replace Array Subset(array=w1242, new element=w1245, index (row)=w1237) -> (w1243:string[][])  [unwired: 1 in]
                  }
                }
                n719 = local write "Save Array"(w1220) -> ()
              }
              frame #12 {
                w1249 = "Trap Density-VT (Traps/Vcm^2):"
                n720 = local read "Save Array"() -> (w1251:string[][])
                n721 = Array Size(array=w1251) -> (size(s)=w1256:i32[])
                n722 = Array Subset(array=w1251, index (row)=0, index (col)=0, length (col)=3) -> (w1252:string[][])  [unwired: 1 in]
                n723 = Index Array(array=w1256, index=0) -> (element=w1258:i32)
                n724 = Reshape Array(w1252, w1258) -> (w1250:string[])
                n725 = Search 1D Array(1D array=w1250, element=w1249) -> (index of element=w1261:i32)  [unwired: 1 in]
                n726 = Equal?(x=w1261, y=-1) -> (x = y?=w1260:bool)
                n727 = case shown="True" w1260 {
                  tunnel: w1251 -> [w1270 w1281]
                  tunnel: w1261 -> [w1268 _]
                  tunnel: [w1267 w1282] -> w1259
                  tunnel: w1250 -> [_ w1280]
                  tunnel: w1249 -> [_ w1279]
                  frame False {
                    n728 = local read "Re-Calculated Values Cluster"() -> (w1265:T9)
                    n729 = Unbundle By Name(w1265) -> ("Trap Density-VT"=w1264:dbl)
                    n730 = Quotient & Remainder(x=w1268, y=3) -> (floor(x/y)=w1263:i32)  [unwired: 1 out]
                    n731 = Format Value(format string="%#g", value (0)=w1264) -> (output string=w1269:string)  [unwired: 1 in]
                    n732 = Replace Array Subset(array=w1270, new element=w1269, index (row)=w1263, index (col)=1) -> (w1267:string[][])
                  }
                  frame True {
                    n733 = local read "Re-Calculated Values Cluster"() -> (w1278:T9)
                    n734 = Unbundle By Name(w1278) -> ("Trap Density-VT"=w1277:dbl)
                    n735 = Search 1D Array(1D array=w1280, element="STS-Sat (V/decade):") -> (index of element=w1274:i32)  [unwired: 1 in]
                    n736 = Add(x=w1274, y=3) -> (x+y=w1273:i32)
                    n737 = Quotient & Remainder(x=w1273, y=3) -> (floor(x/y)=w1276:i32)  [unwired: 1 out]
                    n738 = Format Value(format string="%#g", value (0)=w1277) -> (output string=w1283:string)  [unwired: 1 in]
                    n739 = Build Array(w1279, w1283) -> (w1287:string[])
                    n740 = Increment(x=w1276) -> (x+1=w1286:i32)
                    n741 = Insert Into Array(array=w1281, index (row)=w1286, new element=w1287) -> (w1282:string[][])  [unwired: 1 in]
                  }
                }
                n742 = local write "Save Array"(w1259) -> ()
              }
              frame #13 {
                w1289 = "Trap Density-STS (Traps/Vcm^2):"
                n743 = local read "Save Array"() -> (w1291:string[][])
                n744 = Array Size(array=w1291) -> (size(s)=w1296:i32[])
                n745 = Array Subset(array=w1291, index (row)=0, index (col)=0, length (col)=3) -> (w1292:string[][])  [unwired: 1 in]
                n746 = Index Array(array=w1296, index=0) -> (element=w1298:i32)
                n747 = Reshape Array(w1292, w1298) -> (w1290:string[])
                n748 = Search 1D Array(1D array=w1290, element=w1289) -> (index of element=w1301:i32)  [unwired: 1 in]
                n749 = Equal?(x=w1301, y=-1) -> (x = y?=w1300:bool)
                n750 = case shown="True" w1300 {
                  tunnel: w1291 -> [w1310 w1321]
                  tunnel: w1301 -> [w1309 _]
                  tunnel: [w1308 w1322] -> w1299
                  tunnel: w1290 -> [_ w1320]
                  tunnel: w1289 -> [_ w1319]
                  frame False {
                    n751 = local read "Re-Calculated Values Cluster"() -> (w1305:T9)
                    n752 = Unbundle By Name(w1305) -> ("Trap Density-STS"=w1304:dbl)
                    n753 = Quotient & Remainder(x=w1309, y=3) -> (floor(x/y)=w1303:i32)  [unwired: 1 out]
                    n754 = Format Value(format string="%#g", value (0)=w1304) -> (output string=w1306:string)  [unwired: 1 in]
                    n755 = Replace Array Subset(array=w1310, new element=w1306, index (row)=w1303, index (col)=1) -> (w1308:string[][])
                  }
                  frame True {
                    n756 = local read "Re-Calculated Values Cluster"() -> (w1318:T9)
                    n757 = Unbundle By Name(w1318) -> ("Trap Density-STS"=w1317:dbl)
                    n758 = Search 1D Array(1D array=w1320, element="Trap Density-VT (Traps/Vcm^2):") -> (index of element=w1314:i32)  [unwired: 1 in]
                    n759 = Add(x=w1314, y=3) -> (x+y=w1313:i32)
                    n760 = Quotient & Remainder(x=w1313, y=3) -> (floor(x/y)=w1316:i32)  [unwired: 1 out]
                    n761 = Format Value(format string="%#g", value (0)=w1317) -> (output string=w1328:string)  [unwired: 1 in]
                    n762 = Build Array(w1319, w1328) -> (w1324:string[])
                    n763 = Increment(x=w1316) -> (x+1=w1325:i32)
                    n764 = Insert Into Array(array=w1321, index (row)=w1325, new element=w1324) -> (w1322:string[][])  [unwired: 1 in]
                  }
                }
                n765 = local write "Save Array"(w1299) -> ()
              }
            }
            n766 = local read "New: Temp"() -> (w851:dbl)
            n767 = local read "New: Width"() -> (w852:dbl)
            n768 = local read "New: Length"() -> (w854:dbl)
            n769 = local read "Index"() -> (w853:string)
            n770 = To Long Integer(number=w851) -> (32bit integer=w868:i32)
            n771 = Number To Decimal String(number=w868) -> (decimal integer string=w863:string)  [unwired: 1 in]
            n772 = To Long Integer(number=w852) -> (32bit integer=w867:i32)
            n773 = To Long Integer(number=w854) -> (32bit integer=w866:i32)
            n774 = Strip Path(path=w850) -> (stripped path=w855:path)  [unwired: 1 out]
            n775 = Number To Decimal String(number=w866) -> (decimal integer string=w861:string)  [unwired: 1 in]
            n776 = Number To Decimal String(number=w867) -> (decimal integer string=w860:string)  [unwired: 1 in]
            n777 = Concatenate Strings("_", w863, "K") -> (w865:string)
            n778 = call "Build Text"("Temp"=w865, "Index"=w853, "Length"=w861, "Width"=w860) -> ("Result"=w859:string)  [unwired: 10 in, 1 out]
            n779 = Path To String(path=w855) -> (string=w857:string)
            n780 = Concatenate Strings(w857, "\\", w859) -> (w858:string)
            n781 = String To Path(string=w858) -> (path=w849:path)
          }
          frame #1 {
            n782 = flat-sequence {
              tunnel: w1332 -> [w1334]
              tunnel: w1331 -> [w1333]
              tunnel: [w1333] -> w1330
              tunnel: w1330 -> [w1340]
              tunnel: w1329 -> [w1339]
              frame #0 {
                n783 = Equal?(x=w1334, y=w1333) -> (x = y?=w1335:bool)
                n784 = case shown="False" w1335 {
                  tunnel: w1334 -> [w1338 _]
                  tunnel: w1333 -> [w1337 _]
                  frame False {
                    n785 = Move(source path=w1338, 9:TRUE, 10:w1337) -> ()  [unwired: 2 in, 3 out]
                  }
                  frame True {
                  }
                }
              }
              frame #1 {
                n786 = local write "Transfer File"(w1340) -> ()
                n787 = call-poly <vilib>:"Write To Spreadsheet File.vi"("2D data"=w1339, "file path (dialog if empty)"=w1340) -> ()  [unwired: 6 in, 1 out]
              }
            }
          }
        }
        n788 = local read "Save Next?"() -> (w835:bool)
        n789 = Cluster To Array(cluster=w840) -> (array=w839:bool[])
        n790 = Boolean Array To Number(Boolean array=w839) -> (number=w838:u32)
        n791 = Equal To 0?(x=w838) -> (x = 0?=w837:bool)
        n792 = case shown="True" w837 {
          tunnel: [MegaAwesome_States."Read Data" w847] -> w836
          tunnel: w835 -> [_ w844]
          frame False {
          }
          frame True {
            n793 = Select(t=MegaAwesome_States."Next File", s=w844, f=MegaAwesome_States."No Event") -> (s? t:f=w847:T2)
          }
        }
      }
      frame "Exit" {
        n794 = disable-structure shown="Disabled" {
          disable-tunnel: [w1344 _] -> _
          disable-tunnel: [w1343 _] -> _
          frame Disabled {
            n795 = flat-sequence {
              tunnel: [w1353] -> w1344
              tunnel: [w1353] -> w1343
              frame #0 {
                w1352 = FALSE
                n796 = property on="Next File" class="Bool (strict)"("Value"=w1352) -> (error out=w1347:errorcluster)  [unwired: 2 in, 1 out]
                n797 = property on="Previous File" class="Bool (strict)"(error in=w1347, "Value"=w1352) -> (error out=w1348:errorcluster)  [unwired: 1 in, 1 out]
                n798 = Request Deallocation(TRUE) -> ()
                n799 = property on="Save" class="Bool (strict)"(error in=w1348, "Value"=w1352) -> (error out=w1349:errorcluster)  [unwired: 1 in, 1 out]
                n800 = property on="Export" class="Bool (strict)"("Value"=w1352) -> ()  [unwired: 2 in, 2 out]
                n801 = property on="Save Next" class="Bool (strict)"(error in=w1349, "Value"=w1352) -> (error out=w1350:errorcluster)  [unwired: 1 in, 1 out]
                n802 = property on="Discard" class="Bool (strict)"(error in=w1350, "Value"=w1352) -> (error out=w1351:errorcluster)  [unwired: 1 in, 1 out]
                n803 = property on="Save Lines" class="Bool (strict)"(error in=w1351, "Value"=w1352) -> ()  [unwired: 1 in, 2 out]
                n804 = property on="Close" class="Bool (strict)"("Value"=w1352) -> ()  [unwired: 2 in, 2 out]
                n805 = property on="Disable Flag" class="Bool (strict)"("Value"=w1352) -> ()  [unwired: 2 in, 2 out]
                n806 = call "IMAQ Dispose"("All Images? (No)"=TRUE) -> ()  [unwired: 5 in, 1 out]
              }
              frame #1 {
                w1353 = MegaAwesome_States."Exit"
              }
            }
          }
          frame Enabled {
          }
        }
        n807 = event shown="[0] Application Instance Close?" {
          selector: _ -> [_]
          dyn-events: _ -> [_]
          timeout: _ -> [_]
          event Application Instance Close? {
            n808 = event-data() -> ()  [unwired: 1 in, 4 out]
            n809 = event-data("Discard?"=TRUE) -> ()  [unwired: 2 in, 1 out]
          }
        }
      }
      frame "Save Lines" {
        n810 = Build Path(base path=w1356, name or relative path="ROI") -> (appended path=w1359:path)
        n811 = call <vilib>:"Check if File or Folder Exists.vi"("path"=w1359) -> ("file or folder exists?"=w1357:bool, "dup path"=w1360:path)  [unwired: 8 in, 1 out]
        n812 = case shown="False" w1357 {
          tunnel: w1360 -> [w1368 w1369]
          tunnel: [w1367 w1369] -> w1364
          frame False {
            n813 = Create Folder(path (use dialog)=w1368) -> (created path=w1367:path)  [unwired: 2 in, 2 out]
          }
          frame True {
          }
        }
        n814 = local read "Index"() -> (w1355:string)
        n815 = property on="Image Out" class="ImageControl"() -> ("ROI"=w1361:T18)  [unwired: 2 in, 2 out]
        n816 = Build Path(base path=w1364, name or relative path=w1355) -> (appended path=w1363:path)
        n817 = Flatten To String(anything=w1361) -> (data string=w1362:string)  [unwired: 3 in, 2 out]
        n818 = Write to Text File(file (use dialog)=w1363, text=w1362) -> ()  [unwired: 2 in, 3 out]
      }
      frame "Export" {
        n819 = flat-sequence {
          tunnel: ["Independant Variable:"] -> w1370
          tunnel: w1371 -> [w1427]
          tunnel: w1370 -> [w1426]
          frame #0 {
            n820 = stacked-sequence {
              tunnel: "Independant Variable:" -> [w1375 w1380 w1385 w1390 w1395 w1400 w1405 w1410 w1415 w1420]
              frame #0 {
                n821 = Equal?(x=w1375, y="Length (um):") -> (x = y?=w1376:bool)
                n822 = case shown="True" w1376 {
                  frame False {
                  }
                  frame True {
                    n823 = local write "X Axis Display Type"("1") -> ()
                    n824 = local write "Opj X Axis"("2") -> ()
                  }
                }
              }
              frame #1 {
                n825 = Equal?(x=w1380, y="Sample Temp (K):") -> (x = y?=w1381:bool)
                n826 = case shown="True" w1381 {
                  frame False {
                  }
                  frame True {
                    n827 = local write "X Axis Display Type"("1") -> ()
                    n828 = local write "Opj X Axis"("1") -> ()
                  }
                }
              }
              frame #2 {
                n829 = Equal?(x=w1385, y="Mobility-Sat (cm^2/Vs):") -> (x = y?=w1386:bool)
                n830 = case shown="True" w1386 {
                  frame False {
                  }
                  frame True {
                    n831 = local write "X Axis Display Type"("2") -> ()
                    n832 = local write "Opj X Axis"("2") -> ()
                  }
                }
              }
              frame #3 {
                n833 = Equal?(x=w1390, y="Mobility-Lin (cm^2/Vs):") -> (x = y?=w1391:bool)
                n834 = case shown="True" w1391 {
                  frame False {
                  }
                  frame True {
                    n835 = local write "X Axis Display Type"("2") -> ()
                    n836 = local write "Opj X Axis"("2") -> ()
                  }
                }
              }
              frame #4 {
                n837 = Equal?(x=w1395, y="On/Off I-Sat:") -> (x = y?=w1396:bool)
                n838 = case shown="True" w1396 {
                  frame False {
                  }
                  frame True {
                    n839 = local write "X Axis Display Type"("2") -> ()
                    n840 = local write "Opj X Axis"("2") -> ()
                  }
                }
              }
              frame #5 {
                n841 = Equal?(x=w1400, y="Off I-Sat (A):") -> (x = y?=w1401:bool)
                n842 = case shown="True" w1401 {
                  frame False {
                  }
                  frame True {
                    n843 = local write "X Axis Display Type"("2") -> ()
                    n844 = local write "Opj X Axis"("2") -> ()
                  }
                }
              }
              frame #6 {
                n845 = Equal?(x=w1405, y="Vt-Sat (V):") -> (x = y?=w1406:bool)
                n846 = case shown="True" w1406 {
                  frame False {
                  }
                  frame True {
                    n847 = local write "X Axis Display Type"("1") -> ()
                    n848 = local write "Opj X Axis"("1") -> ()
                  }
                }
              }
              frame #7 {
                n849 = Equal?(x=w1410, y="STS-Sat (V/decade):") -> (x = y?=w1411:bool)
                n850 = case shown="True" w1411 {
                  frame False {
                  }
                  frame True {
                    n851 = local write "Opj X Axis"("1") -> ()
                    n852 = local write "X Axis Display Type"("1") -> ()
                  }
                }
              }
              frame #8 {
                n853 = Equal?(x=w1415, y="Trap Density-VT (Traps/Vcm^2):") -> (x = y?=w1416:bool)
                n854 = case shown="True" w1416 {
                  frame False {
                  }
                  frame True {
                    n855 = local write "X Axis Display Type"("2") -> ()
                    n856 = local write "Opj X Axis"("2") -> ()
                  }
                }
              }
              frame #9 {
                n857 = Equal?(x=w1420, y="Trap Density-STS (Traps/Vcm^2):") -> (x = y?=w1421:bool)
                n858 = case shown="True" w1421 {
                  frame False {
                  }
                  frame True {
                    n859 = local write "X Axis Display Type"("2") -> ()
                    n860 = local write "Opj X Axis"("2") -> ()
                  }
                }
              }
            }
          }
          frame #1 {
            n861 = local read "Transfer Folder"() -> (w1431:path)
            n862 = Build Path(base path=w1431, name or relative path="Stats") -> (appended path=w1432:path)
            n863 = call <vilib>:"Check if File or Folder Exists.vi"("path"=w1432) -> ("file or folder exists?"=w1446:bool, "dup path"=w1445:path)  [unwired: 8 in, 1 out]
            n864 = call "OA_ConnectToOrigin.vi"() -> ("error out"=w1443:errorcluster, "Origin.IOApplication"=w1444:refnum<k7>)  [unwired: 8 in]
            n865 = case shown="False" w1446 {
              tunnel: w1445 -> [w1619 w1620]
              tunnel: [w1618 w1620] -> w1430
              frame False {
                n866 = Create Folder(path (use dialog)=w1619) -> (created path=w1618:path)  [unwired: 2 in, 2 out]
              }
              frame True {
              }
            }
            n867 = call "File Dialog"("start path"=w1432) -> ("selected path"=w1434:path)  [unwired: 11 in, 3 out]
            n868 = call "OA_Load.vi"("error in (no error)"=w1443, "Path"=w1427, "Origin.IOApplication"=w1444) -> ("error out"=w1441:errorcluster, "Origin.IOApplication"=w1442:refnum<k7>)  [unwired: 1 out]
            n869 = call "OAExecute.vi"("script"="document -m 3;", "Error IO"=w1441, "Origin.IOApplication"=w1442) -> ("Error IO Out"=w1439:errorcluster, "Origin.IOApplication"=w1440:refnum<k7>)  [unwired: 1 in, 1 out]
            n870 = stacked-sequence {
              tunnel: w1431 -> [w1457 w1487 w1499 w1521 w1541 w1562 w1583 w1606]
              tunnel: w1430 -> [w1458 w1486 w1500 w1520 w1542 w1563 w1584 w1607]
              tunnel: w1440 -> [w1460 w1484 w1502 w1523 w1544 w1565 w1586 w1609]
              tunnel: w1439 -> [w1459 w1485 w1501 w1522 w1543 w1564 w1585 w1608]
              tunnel: [_ _ _ _ _ _ _ w1604] -> w1429
              tunnel: [_ _ _ _ _ _ _ w1605] -> w1428
              tunnel: w1426 -> [w1456 w1477 w1498 w1519 w1540 w1561 w1582 w1603]
              frame #0 {
                n871 = local read "X Axis Display Type"() -> (w1448:string)
                n872 = local read "Opj X Axis"() -> (w1453:string)
                n873 = Concatenate Strings("window -a MOBLGraph;\nlayer.x.type=", w1453, "; layer.x.label.numFormat = ", w1448, "; Y3 = 1; X3 = 1;", "window -a MOBLTable;\nwindow -s TV;") -> (w1451:string)
                n874 = call "Param_Analysis_7_24b_JW.vi"("Independant Variable"=w1456, "error in (no error)"=w1459, "Data Folder"=w1457, "Parameter String"="Mobility-Lin (cm^2/Vs):", "Parameter Name"="Mobility-Lin", "Stats Folder"=w1458) -> ("error out"=w1462:errorcluster, "Output Array"=w1464:string[][], "Variables"=w1455:T28)  [unwired: 2 in, 1 out]
                n875 = call "Origin_Export_7_27a_JW.vi"("Input Conditions"=w1455, "Analysis Array"=w1464, "error in (no error)"=w1462, "Parameter Worksheet Name"="[MOBLTable]Mobilities", "Parameter Folder Script"="pe_cd \"Mobility-Lin\";", "Origin.IOApplication"=w1460) -> ("error out"=w1461:errorcluster, "reference out"=w1463:refnum<k7>)  [unwired: 3 in, 1 out]
                n876 = call "OAExecute.vi"("script"=w1451, "Error IO"=w1461, "Origin.IOApplication"=w1463) -> ()  [unwired: 1 in, 3 out]
              }
              frame #1 {
                n877 = local read "X Axis Display Type"() -> (w1469:string)
                n878 = local read "Opj X Axis"() -> (w1474:string)
                n879 = Concatenate Strings("window -a MOBSGraph;\nlayer.x.type=", w1474, "; layer.x.label.numFormat = ", w1469, "; Y3 = 1; X3 = 1;", "window -a MOBSTable;\nwindow -s TV;") -> (w1472:string)
                n880 = call "Param_Analysis_7_24b_JW.vi"("Independant Variable"=w1477, "error in (no error)"=w1485, "Data Folder"=w1487, "Parameter String"="Mobility-Sat (cm^2/Vs):", "Parameter Name"="Mobility-Sat", "Stats Folder"=w1486) -> ("error out"=w1480:errorcluster, "Output Array"=w1478:string[][], "Variables"=w1476:T28)  [unwired: 2 in, 1 out]
                n881 = call "Origin_Export_7_27a_JW.vi"("Input Conditions"=w1476, "Analysis Array"=w1478, "error in (no error)"=w1480, "Parameter Worksheet Name"="[MOBSTable]Mobilities", "Parameter Folder Script"="pe_cd \"Mobility-Sat\";", "Origin.IOApplication"=w1484) -> ("error out"=w1479:errorcluster, "reference out"=w1481:refnum<k7>)  [unwired: 3 in, 1 out]
                n882 = call "OAExecute.vi"("script"=w1472, "Error IO"=w1479, "Origin.IOApplication"=w1481) -> ()  [unwired: 1 in, 3 out]
              }
              frame #2 {
                n883 = local read "X Axis Display Type"() -> (w1490:string)
                n884 = local read "Opj X Axis"() -> (w1495:string)
                n885 = Concatenate Strings("window -a NSTSGraph;\nlayer.x.type=", w1495, "; layer.x.label.numFormat = ", w1490, "; Y3 = 1; X3 = 1;", "window -a NSTSTable;\nwindow -s TV;") -> (w1493:string)
                n886 = call "Param_Analysis_7_24b_JW.vi"("Independant Variable"=w1498, "error in (no error)"=w1501, "Data Folder"=w1499, "Parameter String"="Trap Density-STS (Traps/Vcm^2):", "Parameter Name"="Trap Density-STS", "Stats Folder"=w1500) -> ("error out"=w1505:errorcluster, "Output Array"=w1503:string[][], "Variables"=w1497:T28)  [unwired: 2 in, 1 out]
                n887 = call "Origin_Export_7_27a_JW.vi"("Input Conditions"=w1497, "Analysis Array"=w1503, "error in (no error)"=w1505, "Parameter Worksheet Name"="[NSTSTable]Trap Densities", "Parameter Folder Script"="pe_cd \"N-STS\";", "Origin.IOApplication"=w1502) -> ("error out"=w1504:errorcluster, "reference out"=w1506:refnum<k7>)  [unwired: 3 in, 1 out]
                n888 = call "OAExecute.vi"("script"=w1493, "Error IO"=w1504, "Origin.IOApplication"=w1506) -> ()  [unwired: 1 in, 3 out]
              }
              frame #3 {
                n889 = local read "X Axis Display Type"() -> (w1511:string)
                n890 = local read "Opj X Axis"() -> (w1516:string)
                n891 = call "Param_Analysis_7_24b_JW.vi"("Independant Variable"=w1519, "error in (no error)"=w1522, "Data Folder"=w1521, "Parameter String"="Trap Density-VT (Traps/Vcm^2):", "Parameter Name"="Trap Density-Vt", "Stats Folder"=w1520) -> ("error out"=w1526:errorcluster, "Output Array"=w1524:string[][], "Variables"=w1518:T28)  [unwired: 2 in, 1 out]
                n892 = Concatenate Strings("window -a NVtGraph;\nlayer.x.type=", w1516, "; layer.x.label.numFormat = ", w1511, "; Y3 = 1; X3 = 1;", "window -a NVtTable;\nwindow -s TV;") -> (w1514:string)
                n893 = call "Origin_Export_7_27a_JW.vi"("Input Conditions"=w1518, "Analysis Array"=w1524, "error in (no error)"=w1526, "Parameter Worksheet Name"="[NVTTable]Trap Densities", "Parameter Folder Script"="pe_cd \"N-Vt\";", "Origin.IOApplication"=w1523) -> ("error out"=w1525:errorcluster, "reference out"=w1527:refnum<k7>)  [unwired: 3 in, 1 out]
                n894 = call "OAExecute.vi"("script"=w1514, "Error IO"=w1525, "Origin.IOApplication"=w1527) -> ()  [unwired: 1 in, 3 out]
              }
              frame #4 {
                n895 = local read "X Axis Display Type"() -> (w1532:string)
                n896 = local read "Opj X Axis"() -> (w1537:string)
                n897 = Concatenate Strings("window -a OffIGraph;\nlayer.x.type=", w1537, "; layer.x.label.numFormat = ", w1532, "; Y3 = 1; X3 = 1;", "window -a OffITable;\nwindow -s TV;") -> (w1535:string)
                n898 = call "Param_Analysis_7_24b_JW.vi"("Independant Variable"=w1540, "error in (no error)"=w1543, "Data Folder"=w1541, "Parameter String"="Off I-Sat (A):", "Parameter Name"="Off I-Sat", "Stats Folder"=w1542) -> ("error out"=w1547:errorcluster, "Output Array"=w1545:string[][], "Variables"=w1539:T28)  [unwired: 2 in, 1 out]
                n899 = call "Origin_Export_7_27a_JW.vi"("Input Conditions"=w1539, "Analysis Array"=w1545, "error in (no error)"=w1547, "Parameter Worksheet Name"="[OffItable]OffCurrents", "Parameter Folder Script"="pe_cd \"OffI-Sat\";", "Origin.IOApplication"=w1544) -> ("error out"=w1546:errorcluster, "reference out"=w1548:refnum<k7>)  [unwired: 3 in, 1 out]
                n900 = call "OAExecute.vi"("script"=w1535, "Error IO"=w1546, "Origin.IOApplication"=w1548) -> ()  [unwired: 1 in, 3 out]
              }
              frame #5 {
                n901 = local read "X Axis Display Type"() -> (w1553:string)
                n902 = local read "Opj X Axis"() -> (w1558:string)
                n903 = Concatenate Strings("window -a OnOffGraph;\nlayer.x.type=", w1558, "; layer.x.label.numFormat = ", w1553, "; Y3 = 1; X3 = 1;", "window -a OnOffTable;\nwindow -s TV;") -> (w1556:string)
                n904 = call "Param_Analysis_7_24b_JW.vi"("Independant Variable"=w1561, "error in (no error)"=w1564, "Data Folder"=w1562, "Parameter String"="On/Off I-Sat:", "Parameter Name"="OnOff Ratio", "Stats Folder"=w1563) -> ("error out"=w1568:errorcluster, "Output Array"=w1566:string[][], "Variables"=w1560:T28)  [unwired: 2 in, 1 out]
                n905 = call "Origin_Export_7_27a_JW.vi"("Input Conditions"=w1560, "Analysis Array"=w1566, "error in (no error)"=w1568, "Parameter Worksheet Name"="[OnOffTable]On/Off Ratios", "Parameter Folder Script"="pe_cd \"OnOff-Ratio\";", "Origin.IOApplication"=w1565) -> ("error out"=w1567:errorcluster, "reference out"=w1569:refnum<k7>)  [unwired: 3 in, 1 out]
                n906 = call "OAExecute.vi"("script"=w1556, "Error IO"=w1567, "Origin.IOApplication"=w1569) -> ()  [unwired: 1 in, 3 out]
              }
              frame #6 {
                n907 = local read "X Axis Display Type"() -> (w1574:string)
                n908 = local read "Opj X Axis"() -> (w1579:string)
                n909 = call "Param_Analysis_7_24b_JW.vi"("Independant Variable"=w1582, "error in (no error)"=w1585, "Data Folder"=w1583, "Parameter String"="STS-Sat (V/decade):", "Parameter Name"="STS-Sat", "Stats Folder"=w1584) -> ("error out"=w1589:errorcluster, "Output Array"=w1587:string[][], "Variables"=w1581:T28)  [unwired: 2 in, 1 out]
                n910 = Concatenate Strings("window -a SGraph;\nlayer.x.type=", w1579, "; layer.x.label.numFormat = ", w1574, "; Y3 = 1; X3 = 1;", "window -a STable;\nwindow -s TV;") -> (w1577:string)
                n911 = call "Origin_Export_7_27a_JW.vi"("Input Conditions"=w1581, "Analysis Array"=w1587, "error in (no error)"=w1589, "Parameter Worksheet Name"="[STable]Threshold Swing", "Parameter Folder Script"="pe_cd \"STS-Sat\";", "Origin.IOApplication"=w1586) -> ("error out"=w1588:errorcluster, "reference out"=w1590:refnum<k7>)  [unwired: 3 in, 1 out]
                n912 = call "OAExecute.vi"("script"=w1577, "Error IO"=w1588, "Origin.IOApplication"=w1590) -> ()  [unwired: 1 in, 3 out]
              }
              frame #7 {
                n913 = local read "X Axis Display Type"() -> (w1595:string)
                n914 = local read "Opj X Axis"() -> (w1600:string)
                n915 = Concatenate Strings("window -a VtGraph;\nlayer.x.type=", w1600, "; layer.x.label.numFormat = ", w1595, "; Y3 = 1; X3 = 1;", "window -a VtTable;\nwindow -s TV;") -> (w1598:string)
                n916 = call "Param_Analysis_7_24b_JW.vi"("Independant Variable"=w1603, "error in (no error)"=w1608, "Data Folder"=w1606, "Parameter String"="Vt-Sat (V):", "Parameter Name"="Vt-Sat", "Stats Folder"=w1607) -> ("error out"=w1612:errorcluster, "Output Array"=w1610:string[][], "Variables"=w1602:T28)  [unwired: 2 in, 1 out]
                n917 = call "Origin_Export_7_27a_JW.vi"("Input Conditions"=w1602, "Analysis Array"=w1610, "error in (no error)"=w1612, "Parameter Worksheet Name"="[VtTable]Threshold Voltages", "Parameter Folder Script"="pe_cd \"Vt-Sat\";", "Origin.IOApplication"=w1609) -> ("error out"=w1611:errorcluster, "reference out"=w1613:refnum<k7>)  [unwired: 3 in, 1 out]
                n918 = call "OAExecute.vi"("script"=w1598, "Error IO"=w1611, "Origin.IOApplication"=w1613) -> ("Error IO Out"=w1604:errorcluster, "Origin.IOApplication"=w1605:refnum<k7>)  [unwired: 1 in, 1 out]
              }
            }
            n919 = Path To String(path=w1434) -> (string=w1433:string)
            n920 = call "OAExecute.vi"("script"="pe_cd /; ", "Error IO"=w1429, "Origin.IOApplication"=w1428) -> ("Error IO Out"=w1435:errorcluster, "Origin.IOApplication"=w1436:refnum<k7>)  [unwired: 1 in, 1 out]
            n921 = call "OASaveProject.vi"("path"=w1433, "Error IO"=w1435, "Origin.IOApplication"=w1436) -> ("Origin.IOApplication"=w1425:refnum<k7>)  [unwired: 2 out]
            n922 = call "OAEndSession.vi"("Origin.IOApplication"=w1425) -> ()  [unwired: 1 in, 3 out]
          }
        }
      }
    }
    "Current State" <- w12
    "Folder Index" <- w11
    n923 = Wait (ms)(milliseconds to wait=u32 50) -> ()  [unwired: 1 out]
    n924 = Equal?(x=w12, y=MegaAwesome_States."Exit") -> (x = y?=w15:bool)
  }
  n925 = disable-structure shown="Disabled" {
    disable-tunnel: w1 -> [w1622 _]
    frame Disabled {
      n926 = call "Close LabView?"("Enable"=w1622) -> ("OK"=w1621:bool)  [unwired: 17 in, 1 out]
      n927 = Quit LabVIEW(quit? (T)=w1621) -> ()
    }
    frame Enabled {
    }
  }
